vi "Keithley24XX_SR830_Lakeshore336_4Probe_Resistance_Measurement_v2_Controller.vi"() -> ()   [LabVIEW 2018]
uses:
  <instrlib>/Keithley 24XX/Keithley 24XX.lvlib
  <instrlib>/Stanford Research 830/Stanford Research 830.lvlib
  <instrlib>/Lake Shore 336/Lake Shore 336.lvlib
  <instrlib>/Stanford Research 830/Public/Data/Read (All Parameters).vi
  <instrlib>/Keithley 24XX/Public/Data/Read (Single Point).vi
panel:
  in  "Output Level (0)":dbl
  in  "Resistance Manual Range":dbl=1.0
  in  "Current Manual Range":dbl=1.0
  in  "Voltage Manual Range":dbl=1.0
  out "Program Information":string
  out "Front / Rear Terminals":string
  in  "Keithley 24XX Settings":T1(tab)
  out "Enabled Sensing\nFunctions":string
  out "Sensing Current Upper Limit":string
  out "Source Mode:":string
  out "Source Amplitude":dbl
  out "Output Impedence Mode":string
  out "4 Probe Senseing":enum16{"OFF", "ON"}(ring)
  in  "Voltage Auto Range":bool caption="Sync Filter Enabled"
  in  "Current Auto Range":bool caption="Sync Filter Enabled"
  in  "Resistance Auto Range":bool caption="Sync Filter Enabled"
  in  "Update Keithley 24XX GS":bool
  in  "Remote Sensing (4 Wire)":bool
  in  "Displayed Measurement (0: Voltage)":u16(ring)=1 items=["Voltage", "Current", "Resistance"]
  in  "Compliance  Level (0.1)":dbl=0.1
  in  "Source Mode  (0: Voltage)":u16(ring) items=["Voltage", "Current"]
  in  "Output Type  (0: Immediate)":u16(ring) items=["Immediate", "Triggered"]
  out "Output On/Off":bool
  out "Total  Program Iterations":i32
  out "Current Program Iteration":i32
  in  "Program Iterations":i32 min=0 step=1
  out "Channel 1 Display":u16(ring) items=["X", "R", "X Noise", "Aux In 1", "Aux In 2"]
  out "Channel 2 Display":u16(ring) items=["Y", "Theta", "Y Noise", "Aux In 3", "Aux In 4"]
  out "Channel 2\nMeasurement":sgl
  out "Ref\nVoltage (V)":sgl
  out "Channel 1\nMeasurement":sgl
  in  "SR830 Settings":T2(tab)
  out "Channel 1 Display With Ratio":u16(ring) items=["None", "Aux In 1", "Aux In 2"]
  out "Channel 2 Display With Ratio":u16(ring) items=["None", "Aux In 3", "Aux In 4"]
  out "Ref. Amp.":dbl
  out "Ref. Harm.":i32
  out "Ref. Phase":dbl
  out "Trigger Source":u16(ring) items=["Internal", "External"]
  out "Ref. Freq.":dbl
  out "Sensitivity":i16(ring)=-1 items=["Auto Gain"=-1, "2 nV/fA"=0, "5 nV/fA"=1, "10 nV/fA"=2, "20 nV/fA"=3, "50 nV/fA"=4, "100 nV/fA"=5, "200 nV/fA"=6, "500 nV/fA"=7, "1 uV/pA"=8, "2 uV/pA"=9, "5 uV/pA"=10, "10 uV/pA"=11, "20 uV/pA"=12, "50 uV/pA"=13, "100 uV/pA"=14, "200 uV/pA"=15, "500 uV/pA"=16, "1 mV/nA"=17, "2 mV/nA"=18, "5 mV/nA"=19, "10 mV/nA"=20, "20 mV/nA"=21, "50 mV/nA"=22, "100 mV/nA"=23, "200 mV/nA"=24, "500 mV/mA"=25, "1 V/uA"=26]
  out "Time Constant":u16(ring)=8 items=["10 us", "30 us", "100 us", "300 us", "1 ms", "3 ms", "10 ms", "30 ms", "100 ms", "300 ms", "1 s", "3 s", "10 s", "30 s", "100 s", "300 s", "1 ks", "3 ks", "10 ks", "30 ks"]
  out "Low Pass Filter Slope":u16(ring)=1 items=["6 dB/oct", "12 dB/oct", "18 db/oct", "24 dB/oct"]
  out "Input Notch Filter":u16(ring) items=["None", "Line Notch", "2x Line Notch", "Both Notch Filters"]
  out "Dynamic Reserve":i16(ring)=-1 items=["Auto Reserve"=-1, "High Reserve"=0, "Normal"=1, "Low Noise"=2]
  out "Sync Filter Enabled":enum16{"False", "True"}(ring)
  out "Input Shield Grounding":u16(ring) items=["Float", "Ground"]
  out "Input Coupling":u16(ring) items=["AC", "DC"]
  out "Input Connection":u16(ring) items=["Single-Ended Voltage", "Differential Voltage", "1 MOhm Current Gain", "100 MOhm Current Gain"]
  in  "Aquire SR830 GS":bool
  in  "Channel 1 Display With Ratio":u16(ring) items=["None", "Aux In 1", "Aux In 2"]
  in  "Channel 2 Display With Ratio":u16(ring) items=["None", "Aux In 3", "Aux In 4"]
  in  "Channel 1 Display":u16(ring) items=["X", "R", "X Noise", "Aux In 1", "Aux In 2"]
  in  "Channel 2 Display":u16(ring)=1 items=["Y", "Theta", "Y Noise", "Aux In 3", "Aux In 4"]
  in  "Dynamic Reserve":i16(ring)=1 items=["Auto Reserve"=-1, "High Reserve"=0, "Normal"=1, "Low Noise"=2]
  in  "Sensitivity":i16(ring)=17 items=["Auto Gain"=-1, "2 nV/fA"=0, "5 nV/fA"=1, "10 nV/fA"=2, "20 nV/fA"=3, "50 nV/fA"=4, "100 nV/fA"=5, "200 nV/fA"=6, "500 nV/fA"=7, "1 uV/pA"=8, "2 uV/pA"=9, "5 uV/pA"=10, "10 uV/pA"=11, "20 uV/pA"=12, "50 uV/pA"=13, "100 uV/pA"=14, "200 uV/pA"=15, "500 uV/pA"=16, "1 mV/nA"=17, "2 mV/nA"=18, "5 mV/nA"=19, "10 mV/nA"=20, "20 mV/nA"=21, "50 mV/nA"=22, "100 mV/nA"=23, "200 mV/nA"=24, "500 mV/mA"=25, "1 V/uA"=26]
  in  "Sync Filter Enabled":bool
  in  "Low Pass Filter Slope":u16(ring)=1 items=["6 dB/oct", "12 dB/oct", "18 db/oct", "24 dB/oct"]
  in  "Time Constant":u16(ring)=9 items=["10 us", "30 us", "100 us", "300 us", "1 ms", "3 ms", "10 ms", "30 ms", "100 ms", "300 ms", "1 s", "3 s", "10 s", "30 s", "100 s", "300 s", "1 ks", "3 ks", "10 ks", "30 ks"]
  in  "Input Notch Filter (0: None)":u16(ring) items=["None", "Line Notch", "2x Line Notch", "Both Notch Filters"]
  in  "Internal Ref. Freq. (Hz)":dbl=17.0 min=1.0 max=19999.0 step=1.0
  in  "Detection Harmonic Num.":dbl=1.0
  in  "Sine Ref Amplitude (V)":dbl=1.0 min=0.004 max=5.0
  in  "Manual Phase (Degree)":dbl min=-179.99 max=180.0
  in  "Trigger Source":u16(ring) items=["Internal", "External"]
  in  "Input Shield Grounding":u16(ring) items=["Float", "Ground"]
  in  "Input Coupling":u16(ring) items=["AC", "DC"]
  in  "Input Connection":u16(ring)=1 items=["Single-Ended Voltage", "Differential Voltage", "1 MOhm Current Gain", "100 MOhm Current Gain"]
  in  "Update SR830 GS":bool
  in  "Num Steps":i32=1 min=1 step=1
  in  "Total Time (s)":dbl=1.0
  out "Reference Voltage":cluster{u32, dbl}[](graph)
  out "Step Size (V)":dbl=1.0 min=0.004 max=5.0
  in  "Start Output Amplitude (V)":dbl=1.0 min=0.004 max=5.0
  in  "Final Output Amplitude (V)":dbl=1.0 min=0.004 max=5.0
  out "Step Time (ms)":dbl=50.0
  in  "Idle Measuring Time (ms)":i32=500
  out "VI State":T3(ring)
  in  "Idle Measure\nLakeShore 336 \nStatus":bool=TRUE
  in  "Idle Measure \nKeithley 24XX\nStatus":bool=TRUE
  in  "Idle Measure\nSR830 Status":bool=TRUE
  in  "Lakeshore 366\nVISA resource name":refnum<visa-resource-name>="GPIB0::12::INSTR"
  in  "Lakeshore Initialized / Off":bool
  in  "Reset LakeShore\non Initialize":bool
  in  "Keithley24XX Gate\nVISA resource name":refnum<visa-resource-name>="GPIB0::23::INSTR" caption="Keithley 24XX Gate\nVISA resource name"
  in  "Keithley 24XX Initialized / Off":bool
  in  "Reset Keithley\non Initialize":bool
  in  "SR830 Initialized / Off":bool
  in  "Reset SR830\non Initialize":bool
  in  "SR830\nVISA resource name":refnum<visa-resource-name>="GPIB0::8::INSTR" caption="SR830 VISA \nresource name"
  out "Theta : XYGraph":cluster{"Y":dbl[], "Y":dbl[]}[](graph)
  out "Temp : XYGraph":cluster{"Y":dbl[], "Y":dbl[]}[](graph)
  out "Resistance : XYGraph":cluster{"Y":dbl[], "Y":dbl[]}[](graph)
  out "I_leak : XYGraph":cluster{"Y":dbl[], "Y":dbl[]}[](graph)
  out "Resistance / Differential":bool
  out "Gate Voltage":bool
  in  "Temperature":bool
  in  "Phase":bool
  in  "Gate Leakage Current":bool
  out "Dup path":path
  in  "<File Name>.txt (Don't add extension)":string
  in  "Data Save Path:":path=path "C:/Users/labpc/Documents/ProbeStation Users Data"
  in  "Measurement Output":T4(radio)
  in  "Series Resistance (Ohms)\n[Apparatus Constant]":dbl=10000000.0 format="%_6e"
  in  "Measurement \nDelay Time (s)":dbl=30.0
  in  "Source Voltage\nStep Time (ms)\n 4Probe":dbl=20.0
  in  "Source Voltage\nStep Size (V) \n4Probe":dbl=0.01
  in  "Source Measurement Voltage (V)":dbl=1.0
  in  "Source Voltage \nWarmup Delay \n(Before Gating)":bool
  in  "Source Voltage\nRamp On/Off":bool
  in  "Source Voltage\nStep Time (ms)":dbl=200.0
  in  "Source Voltage\nStep Size (V)":dbl=0.05
  in  "Source Voltage\nFinal (V)":dbl
  in  "Source Voltage\nInitial (V)":dbl
  out "Measured Gate\nVoltage (V)":sgl
  out "Gate leakage \ncurrent (A)":sgl
  in  "Gate\nMeasure":bool
  in  "Gate \nStep Time (ms)":dbl=200.0
  in  "Gate\nStep Time (ms)":dbl=200.0
  in  "Gate Voltage\nStep Size (V)":dbl=0.05
  in  "Gate \nVoltage Final (V)":dbl
  in  "Low Gate \nVoltage (V)":dbl=-80.0
  in  "Gate Voltage\nInitial Traversal Direction":enum16{"Upward", "Downward"}(ring)
  in  "Gate Voltage \nStep Size (V)":dbl=0.1
  in  "High Gate \nVoltage (V)":dbl=80.0
  in  "Gate Voltage\nInitial (V)":dbl
  in  "Gate\nReset":bool
  in  "Gate Current\nCompliance Level (A)":dbl=1.0000000005838672e-07
  in  "Run Program":bool
  in  "Stop VI":bool
  in  "Program Selection":T5(radio)
  # "Welcome to Matt Gebert's Keithley / SR830 / Lakeshore 4 Probe Measurement Controller. This Labview program controls the configuration and measurements of one Keithelys 24XX, one SR830 and one LakeShore Controller, through a state machine architecture.\nIf using sensitive samples, be careful of \"rsetting\" equipment, due to fluctuations of output signals. \"General settings\" tabs will be applied at the start of a measurement program, or by being manually applied (button on page).\nPrograms written allow:\n   1) Ramp voltages to initial points for measurements.     2) Perform a 4 Probe DC Gate measurement using the Keithley & SR830."
  # "Sensing Configuration"
  # "Program: Ramp Gate Voltage Configuration"
  # "Program Control"
  # "Program: 4 Probe Measurement Configuration"
  # "Input Configuration"
  # "Measurement Configuration"
  # "Reference Configuration"
  # "Channel Displays"
  # "Channel Displays"
  # "Reference Configuration"
  # "Input Configuration"
  # "Measurement Configuration"
  # "Ramps source voltage to avoid damaging samples.\nNote the current Ref Voltage above if you are in the \"Idle\" state."
  # "4 Probe Output Configuration"
  # "Recorded Params"
  # "Output Data"
  # "Program: 4 Probe Measurement Configuration"
  # "Program: Ramp Source Voltage Configuration"
  # "SR830 Source\n& Meas. Control"
  # "Keithley Gate\nVoltage Control"
  # "LakeShore 336 \nTemperature \nController"
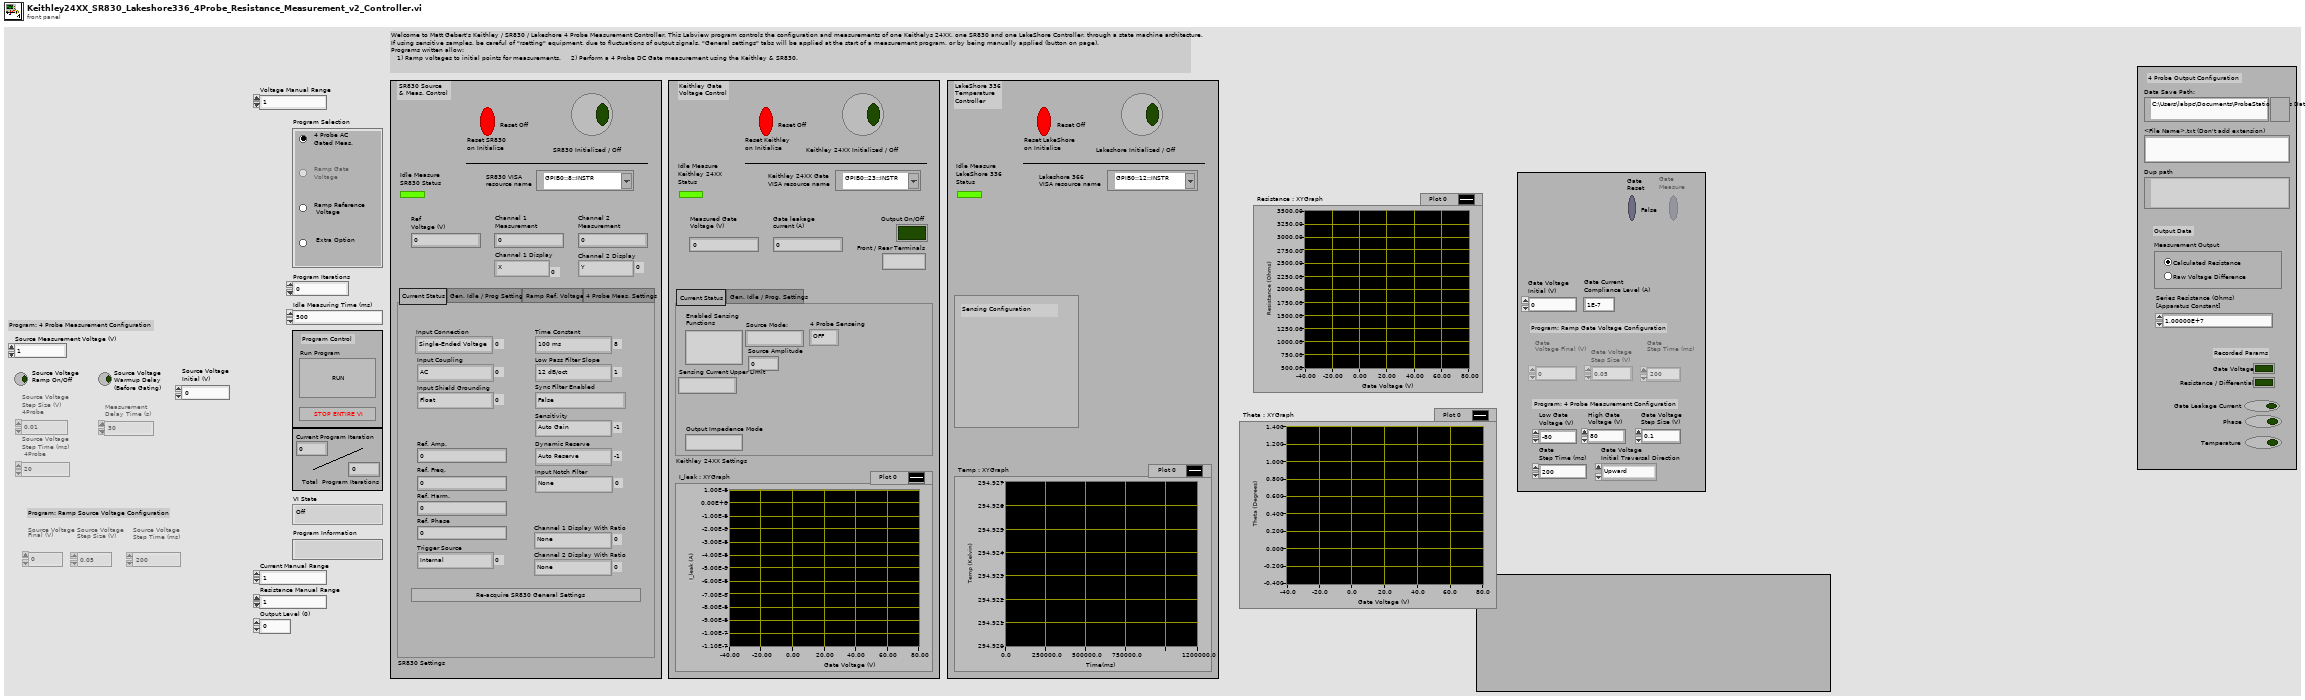
[diagram p1: front panel]
types:
  T1 = enum32{"Current Status", "Gen. Idle / Prog. Settings"}
  T2 = enum32{"Current Status", "Gen. Idle / Prog Settings", "Ramp Ref. Voltage", "4 Probe Meas. Settings"}
  T3 = enum16{"Off", "Idle | Waiting for event", "Running single meas.", "Running multi meas.", "Running continuous meas."}
  T4 = enum32{"Calculated Resistance", "Raw Voltage Difference"}
  T5 = enum32{"4 Probe Gated Measurement", "Ramp Gate Voltage", "Ramp Ref Voltage", "Extra Option"}
  T6 = enum32{"Current Status", "Gen. Idle / Prog. Settings", "Ramp Ref. Voltage", "4 Probe Meas. Settings"}
  T7 = cluster{"Lakeshore 366 VISA Name":refnum<visa-resource-name>, "Lakeshore Error":errorcluster, "Keithley 24XX VISA Name":refnum<visa-resource-name>, "Keithley 24XX Error":errorcluster, "SR830 VISA Name":refnum<visa-resource-name>, "SR830 Error":errorcluster, "MeasurementsRemaining":i32, "TotalMeasurements":i32}
  T8 = cluster{"Baud Rate":u32, "Parity":u16, "Data Bits":u16, "Stop Bits":u16, "Flow Control":u16}
  T9 = cluster{"X-Value":dbl, "Y-Value":dbl, "R-Value":dbl, "Theta-Value":dbl, "Aux In 1 Value":dbl, "Aux In 2 Value":dbl, "Aux In 3 Value":dbl, "Aux In 4 Value":dbl, "Reference Frequency":dbl, "Channel 1 Display":dbl, "Channel 2 Display":dbl}
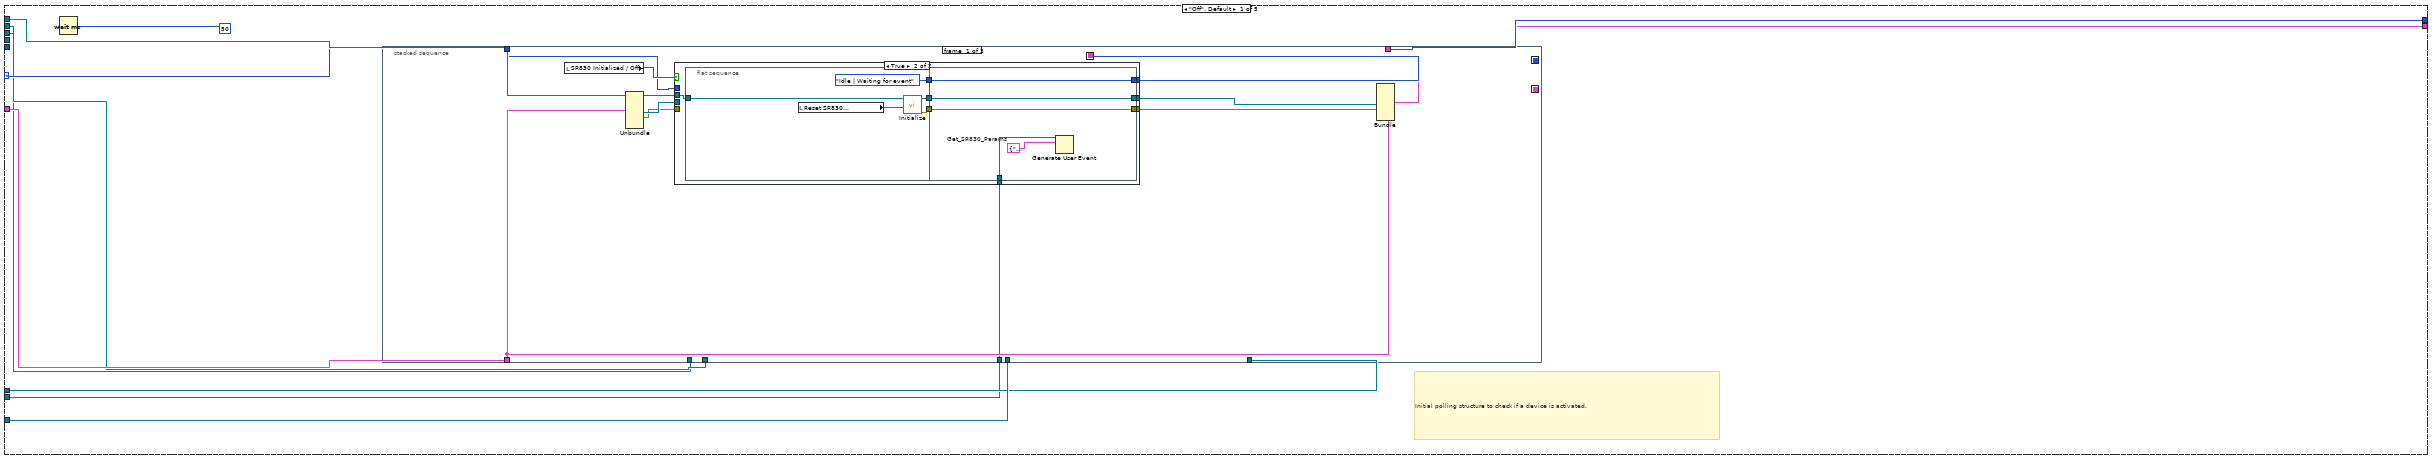
[diagram p7: hidden frame]
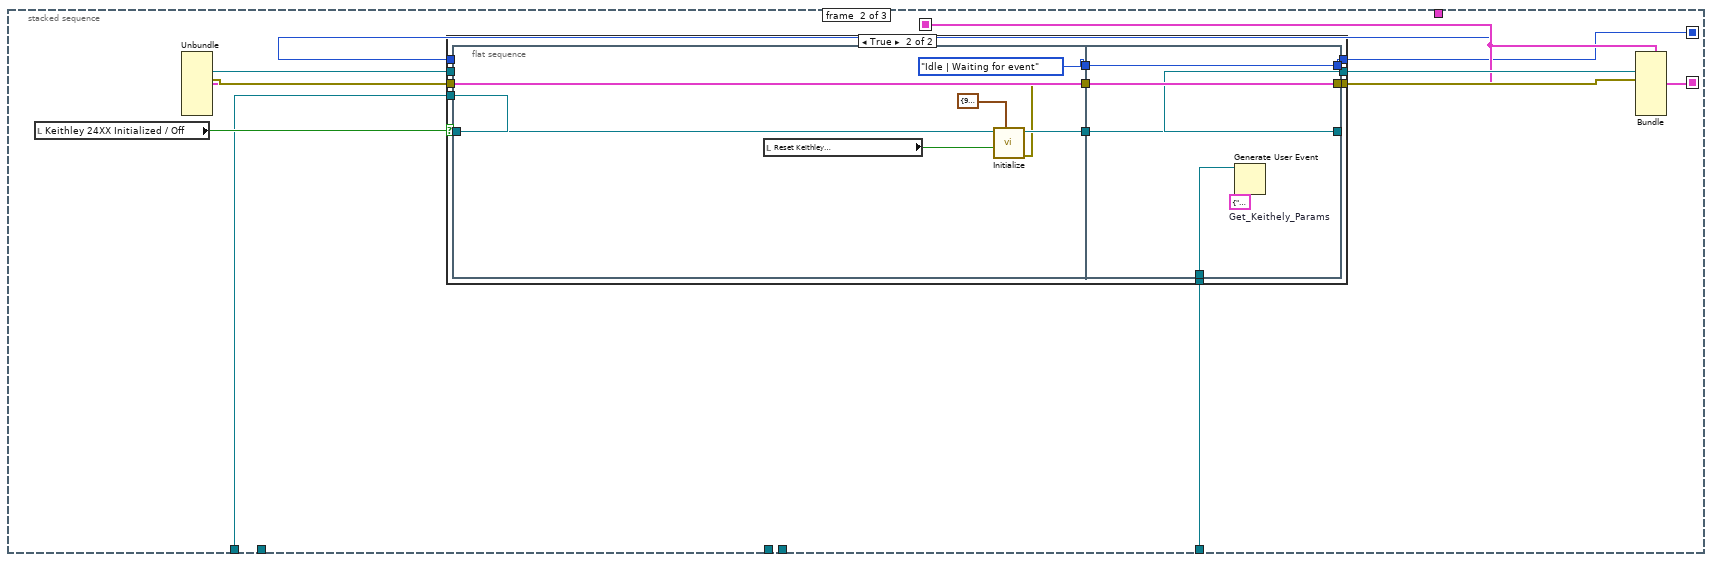
[diagram p9: hidden frame]
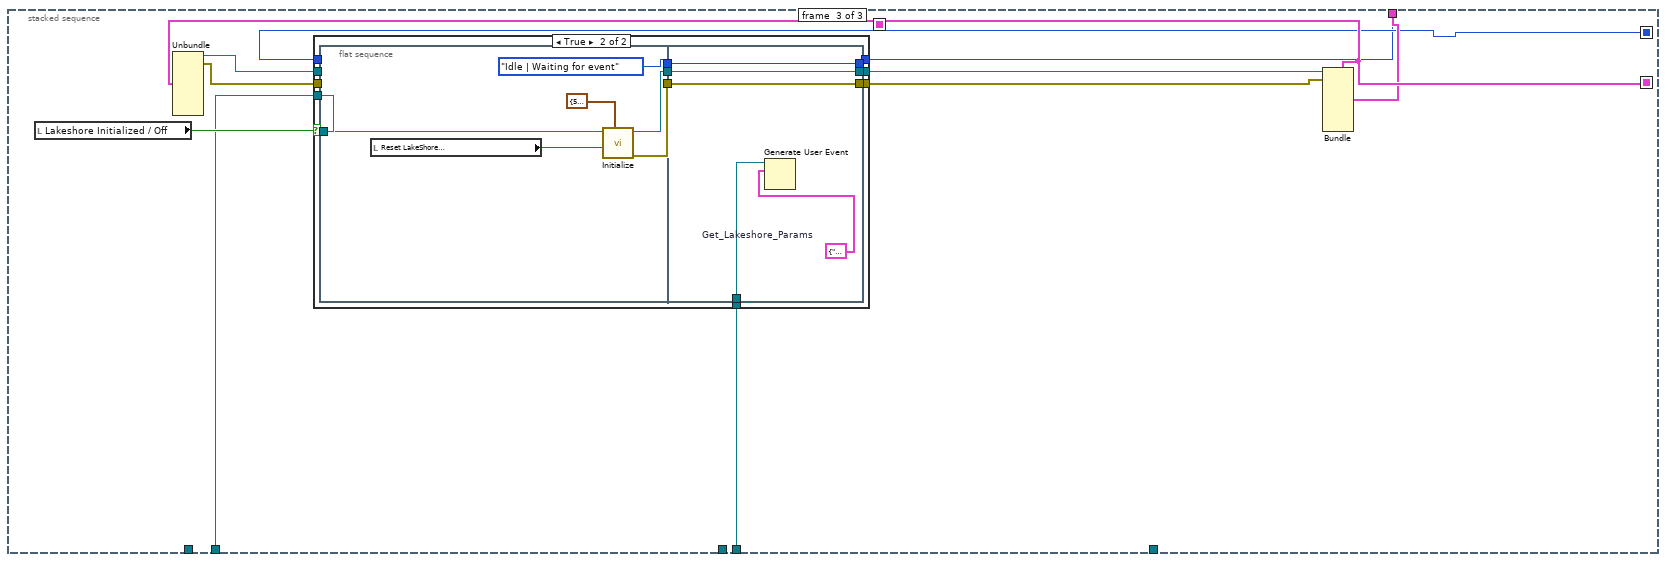
[diagram p11: hidden frame]
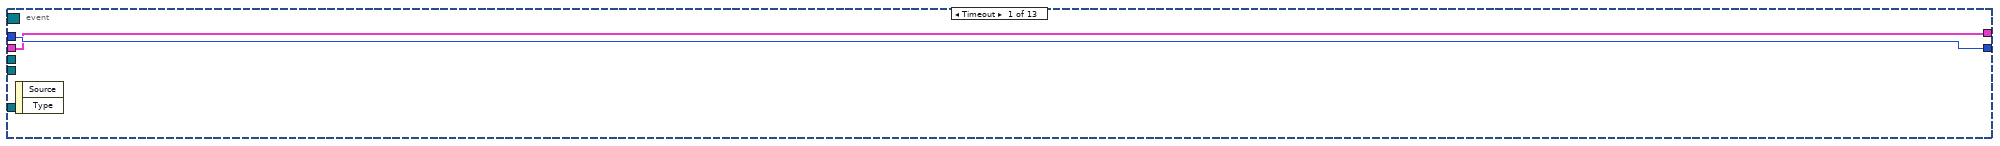
[diagram p13: hidden frame]
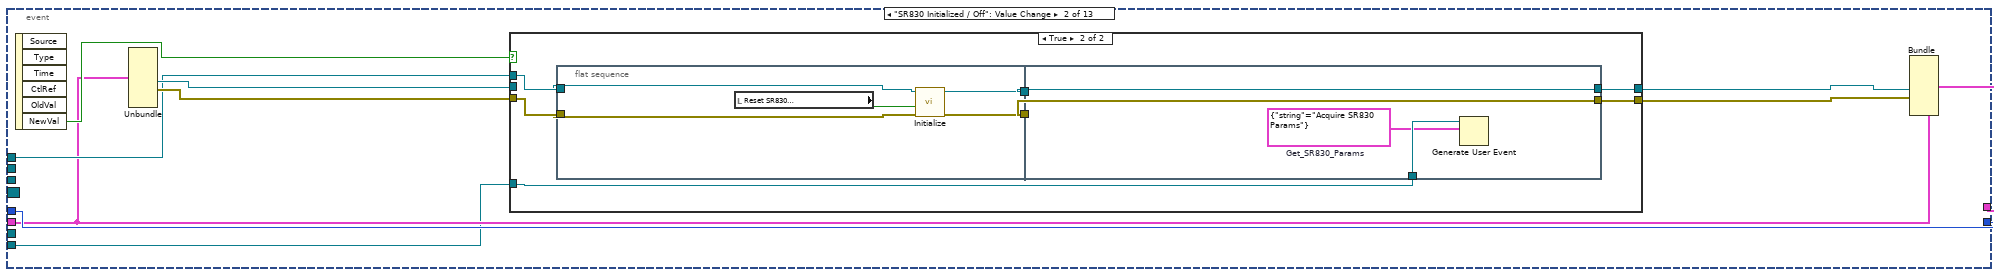
[diagram p14: hidden frame]
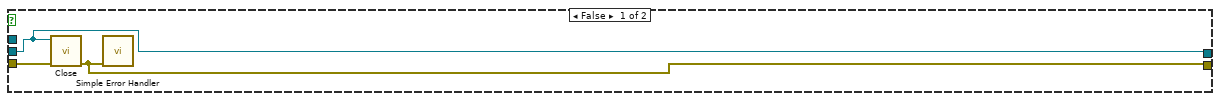
[diagram p15: hidden frame]
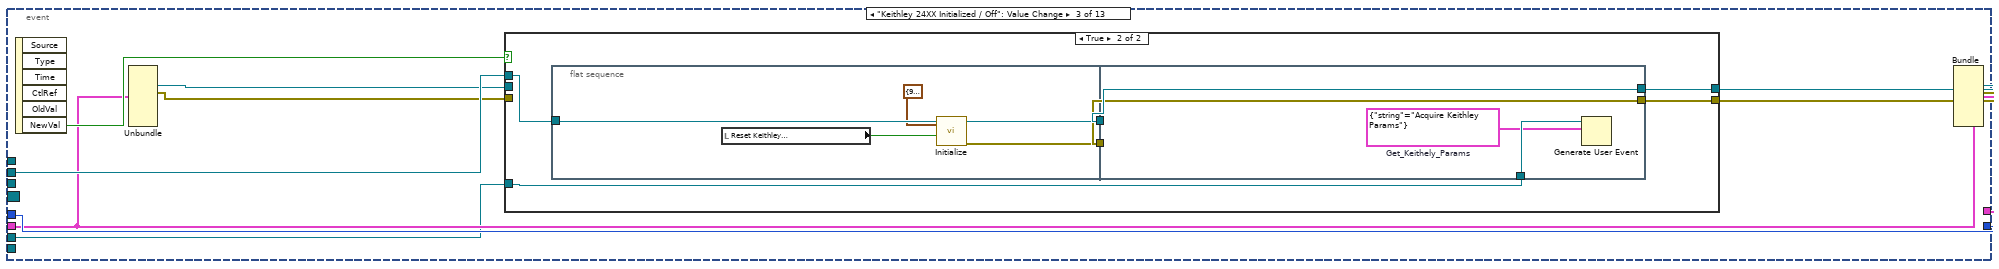
[diagram p16: hidden frame]
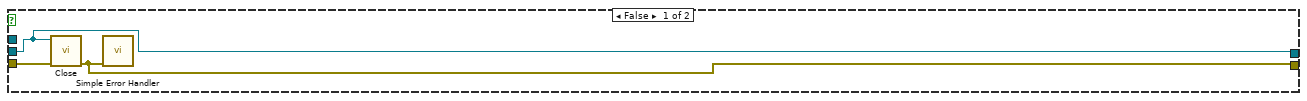
[diagram p17: hidden frame]
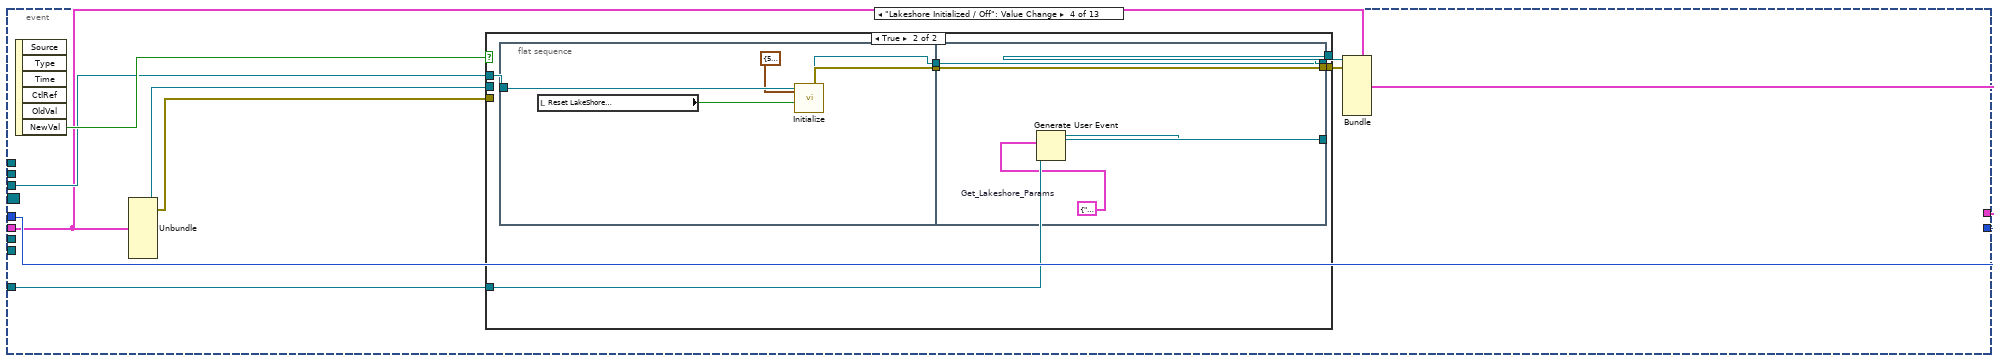
[diagram p18: hidden frame]
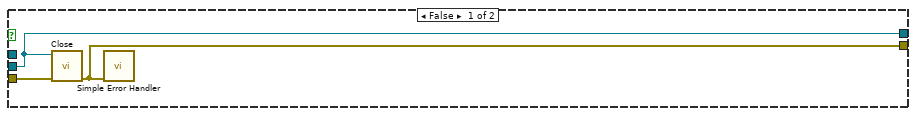
[diagram p19: hidden frame]
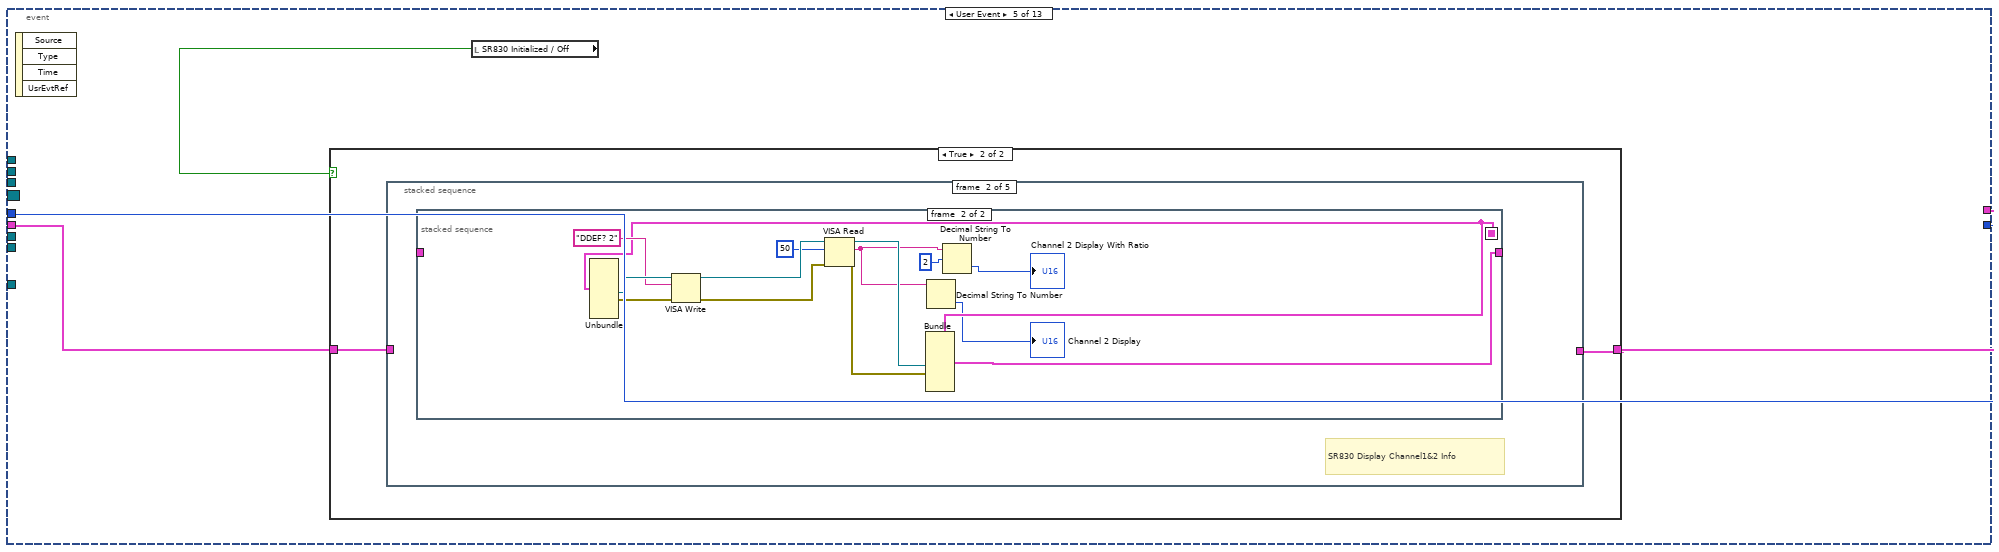
[diagram p20: hidden frame]
diagram:
  w7 = cluster{"string":string} {"string"="Acquire Lakeshore Params"}  # Get_Lakeshore_Params
  w4 = cluster{"string":string} {"string"="Acquire SR830 Params"}  # Get_SR830_Params
  w8 = cluster{"string":string} {"string"="Acquire Keithley Params"}  # Get_Keithely_Params
  w9 = cluster{"string":string} {"string"="UI Update"}  # UI Update
  (unwired) T6."Current Status" ("SR830 Settings")
  w12 = FALSE ("Lakeshore Initialized / Off")
  w19 = TRUE ("Gate Voltage")
  # "TODO: \n1. Make resource error checking mechanism for programs and Idle loop.\n2. Figure out why exiting loop doesn't display generated errors...\n4. Add radio buttons for a) continuous, b) multiple, c) single measurements\n3. UI updates for changing \"Program Selection\" value. Ie, which measurement types are allowed.\n4. UI Updates for enabling / disabling resources\n5. Program event data changes for ramping"
  # "Ensure devices are disconnected on program exit, if \"stopped\"."
  n1 = local read "SR830 Settings"() -> ()  [unwired: 1 in]
  n2 = Create User Event(user event datatype=w9) -> (user event=w5:refnum<user-event>)  [unwired: 1 in, 1 out]
  n3 = Create User Event(user event datatype=w7) -> (user event=w1:refnum<user-event>)  [unwired: 1 in, 1 out]
  n4 = Create User Event(user event datatype=w8) -> (user event=w2:refnum<user-event>)  [unwired: 1 in, 1 out]
  n5 = Create User Event(user event datatype=w4) -> (user event=w3:refnum<user-event>)  [unwired: 1 in, 1 out]
  n6 = register-events(w5, w2, w3, w1) -> (reference out=w6:refnum<event-registration>)  [unwired: 2 in, 1 out]
  n7 = local write "SR830 Initialized / Off"(w12) -> ()
  n8 = local write "Keithley 24XX Initialized / Off"(w12) -> ()
  n9 = local write "Lakeshore Initialized / Off"(w12) -> ()
  n10 = while {
    shift-right: [w29] -> w15
    shift-left: T3."Off" -> [w32]
    shift-right: [w25] -> w13
    shift-left: T7 {"Lakeshore 366 VISA Name"="", "Lakeshore Error"={"status"=FALSE, "code"=0, "source"=""}, "Keithley 24XX VISA Name"="", "Keithley 24XX Error"={"status"=FALSE, "code"=0, "source"=""}, "SR830 VISA Name"="", "SR830 Error"={"status"=FALSE, "code"=0, "source"=""}, "MeasurementsRemaining"=0, "TotalMeasurements"=0} -> [w26]
    tunnel: "Program Selection" -> [w24]
    tunnel: w6 -> [w23]
    tunnel: w3 -> [w22]
    tunnel: w2 -> [w21]
    tunnel: w1 -> [w20]
    stop <- "Stop VI" stop-if-true
    # "State Machine"
    n11 = local read "Keithley24XX Gate\nVISA resource name"() -> (w31:refnum<visa-resource-name>)
    n12 = local read "Lakeshore 366\nVISA resource name"() -> (w30:refnum<visa-resource-name>)
    n13 = local read "SR830\nVISA resource name"() -> (w27:refnum<visa-resource-name>)
    n14 = case shown="\"Idle | Waiting for event\"" w32 {
      selector: w32 -> [w42 w158 _ w908 w918]
      tunnel: w31 -> [w37 w153 _ _ _]
      tunnel: w30 -> [w38 w155 _ _ _]
      tunnel: [w41 w157 T3."Idle | Waiting for event" w907 w918] -> w29
      tunnel: w27 -> [w43 w154 _ _ _]
      tunnel: w26 -> [w40 w152 w878 w910 w917]
      tunnel: [w39 w147 w879 w904 w917] -> w25
      tunnel: w24 -> [_ _ w880 _ _]
      tunnel: w23 -> [_ w145 _ _ _]
      tunnel: w22 -> [w33 w144 _ _ _]
      tunnel: w21 -> [w34 w143 _ _ _]
      tunnel: w20 -> [w35 w142 _ _ _]
      frame "Off", Default {
        # "Initial polling structure to check if a device is activated."
        n15 = Wait (ms)(milliseconds to wait=u32 50) -> ()  [unwired: 1 out]
        n16 = stacked-sequence {
          seq-local: [w47 _ _] -> [_ w81 _]
          seq-local: [w45 _ _] -> [_ w82 _]
          seq-local: [_ w80 _] -> [_ _ w111]
          seq-local: [_ w78 _] -> [_ _ w114]
          tunnel: w43 -> [w49 _ _]
          tunnel: w42 -> [w48 _ _]
          tunnel: w40 -> [w46 _ _]
          tunnel: w37 -> [_ w77 _]
          tunnel: [_ _ w110] -> w41
          tunnel: [_ _ w113] -> w39
          tunnel: w38 -> [_ _ w112]
          tunnel: w35 -> [_ _ w109]
          tunnel: w34 -> [_ w76 _]
          tunnel: w33 -> [w44 _ _]
          frame #0 {
            n17 = local read "SR830 Initialized / Off"() -> (w54:bool)
            n18 = Unbundle(w46) -> ("SR830 VISA Name"=w51:refnum<visa-resource-name>, "SR830 Error"=w50:errorcluster)  [unwired: 6 out]
            n19 = case shown="True" w54 {
              tunnel: w49 -> [_ w65]
              tunnel: [w57 w64] -> w53
              tunnel: [w55 w63] -> w52
              tunnel: w51 -> [w57 _]
              tunnel: w50 -> [w55 _]
              tunnel: w48 -> [w56 _]
              tunnel: [w56 w62] -> w47
              tunnel: w44 -> [_ w58]
              frame False {
              }
              frame True {
                n20 = flat-sequence {
                  tunnel: w65 -> [w70]
                  tunnel: [w69] -> w61
                  tunnel: [w68] -> w60
                  tunnel: [T3."Idle | Waiting for event"] -> w59
                  tunnel: [w73] -> w62
                  tunnel: [w74] -> w63
                  tunnel: [w75] -> w64
                  tunnel: w61 -> [w75]
                  tunnel: w60 -> [w74]
                  tunnel: w59 -> [w73]
                  tunnel: w58 -> [w71]
                  frame #0 {
                    n21 = local read "Reset SR830\non Initialize"() -> (w67:bool)
                    n22 = call <instrlib>:"Initialize.vi"("Reset (True)"=w67, "VISA resource name"=w70) -> ("error out"=w68:errorcluster, "VISA resource name out"=w69:refnum<visa-resource-name>)  [unwired: 8 in]
                  }
                  frame #1 {
                    w72 = cluster{"string":string} {"string"="Acquire SR830 Params"}  # Get_SR830_Params
                    n23 = Generate User Event(user event=w71, event data cluster=w72) -> ()  [unwired: 2 in, 2 out]
                  }
                }
              }
            }
            n24 = Bundle(cluster=w46, "SR830 VISA Name"=w53, "SR830 Error"=w52) -> (w45:T7)  [unwired: 6 in]
          }
          frame #1 {
            n25 = local read "Keithley 24XX Initialized / Off"() -> (w79:bool)
            n26 = Unbundle(w82) -> ("Keithley 24XX VISA Name"=w83:refnum<visa-resource-name>, "Keithley 24XX Error"=w84:errorcluster)  [unwired: 6 out]
            n27 = case shown="True" w79 {
              tunnel: [w87 w96] -> w86
              tunnel: [w89 w97] -> w85
              tunnel: w83 -> [w89 _]
              tunnel: w84 -> [w87 _]
              tunnel: [w88 w95] -> w80
              tunnel: w81 -> [w88 _]
              tunnel: w77 -> [_ w94]
              tunnel: w76 -> [_ w90]
              frame False {
              }
              frame True {
                n28 = flat-sequence {
                  tunnel: w94 -> [w98]
                  tunnel: [w103] -> w93
                  tunnel: [w102] -> w92
                  tunnel: [T3."Idle | Waiting for event"] -> w91
                  tunnel: [w106] -> w95
                  tunnel: [w107] -> w96
                  tunnel: [w108] -> w97
                  tunnel: w93 -> [w108]
                  tunnel: w92 -> [w107]
                  tunnel: w91 -> [w106]
                  tunnel: w90 -> [w104]
                  frame #0 {
                    n29 = local read "Reset Keithley\non Initialize"() -> (w100:bool)
                    n30 = call <instrlib>:"Initialize.vi"("Serial Configuration"=T8 {"Baud Rate"=9600, "Parity"=0, "Data Bits"=8, "Stop Bits"=10, "Flow Control"=0}, "Reset (True)"=w100, "VISA resource name"=w98) -> ("error out"=w102:errorcluster, "VISA resource name out"=w103:refnum<visa-resource-name>)  [unwired: 7 in]
                  }
                  frame #1 {
                    w105 = cluster{"string":string} {"string"="Acquire Keithley Params"}  # Get_Keithely_Params
                    n31 = Generate User Event(user event=w104, event data cluster=w105) -> ()  [unwired: 2 in, 2 out]
                  }
                }
              }
            }
            n32 = Bundle(cluster=w82, "Keithley 24XX VISA Name"=w85, "Keithley 24XX Error"=w86) -> (w78:T7)  [unwired: 6 in]
          }
          frame #2 {
            n33 = local read "Lakeshore Initialized / Off"() -> (w115:bool)
            n34 = Unbundle(w114) -> ("Lakeshore 366 VISA Name"=w116:refnum<visa-resource-name>, "Lakeshore Error"=w117:errorcluster)  [unwired: 6 out]
            n35 = case shown="True" w115 {
              tunnel: [w121 w130] -> w119
              tunnel: [w122 w129] -> w118
              tunnel: w116 -> [w122 _]
              tunnel: w117 -> [w121 _]
              tunnel: [w120 w128] -> w110
              tunnel: w112 -> [_ w127]
              tunnel: w111 -> [w120 _]
              tunnel: w109 -> [_ w123]
              frame False {
              }
              frame True {
                n36 = flat-sequence {
                  tunnel: w127 -> [w131]
                  tunnel: [w135] -> w126
                  tunnel: [w134] -> w125
                  tunnel: [T3."Idle | Waiting for event"] -> w124
                  tunnel: [w139] -> w128
                  tunnel: [w140] -> w129
                  tunnel: [w141] -> w130
                  tunnel: w126 -> [w141]
                  tunnel: w125 -> [w140]
                  tunnel: w124 -> [w139]
                  tunnel: w123 -> [w137]
                  frame #0 {
                    n37 = local read "Reset LakeShore\non Initialize"() -> (w133:bool)
                    n38 = call <instrlib>:"Initialize.vi"("Serial Configuration"=T8 {"Baud Rate"=57600, "Parity"=1, "Data Bits"=7, "Stop Bits"=10, "Flow Control"=0}, "Reset (True)"=w133, "VISA resource name"=w131) -> ("error out"=w135:errorcluster, "VISA resource name out"=w134:refnum<visa-resource-name>)  [unwired: 7 in]
                  }
                  frame #1 {
                    w138 = cluster{"string":string} {"string"="Acquire Lakeshore Params"}  # Get_Lakeshore_Params
                    n39 = Generate User Event(user event=w137, event data cluster=w138) -> ()  [unwired: 2 in, 2 out]
                  }
                }
              }
            }
            n40 = Bundle(cluster=w114, "Lakeshore 366 VISA Name"=w118, "Lakeshore Error"=w119) -> (w113:T7)  [unwired: 6 in]
          }
        }
      }
      frame "Idle | Waiting for event" {
        n41 = flat-sequence {
          tunnel: w158 -> [w170]
          tunnel: [w169] -> w156
          tunnel: w155 -> [w168]
          tunnel: w154 -> [w167]
          tunnel: w153 -> [w166]
          tunnel: w152 -> [w165]
          tunnel: [w164] -> w148
          tunnel: w145 -> [w162]
          tunnel: w144 -> [w161]
          tunnel: w143 -> [w160]
          tunnel: w142 -> [w159]
          tunnel: w156 -> [w804]
          tunnel: [w805] -> w151
          tunnel: [w803] -> w150
          tunnel: [w802] -> w149
          tunnel: [w801] -> w146
          tunnel: [w815] -> w157
          tunnel: w151 -> [w815]
          tunnel: w150 -> [w811]
          tunnel: w149 -> [w810]
          tunnel: w148 -> [w814]
          tunnel: [w813] -> w147
          tunnel: w146 -> [w812]
          frame #0 {
            n42 = event shown="[11] \"Update Keithley 24XX GS\": Mouse Up" {
              selector: w162 -> [_ _ _ _ _ _ _ _ _ _ _ _ _]
              dyn-events: _ -> [_ _ _ _ _ _ _ _ _ _ _ _ _]
              timeout: "Idle Measuring Time (ms)" -> [_ _ _ _ _ _ _ _ _ _ _ _ _]
              tunnel: w170 -> [w172 w176 w205 w238 w258 w481 w584 w586 w588 _ w612 w715 w793]
              tunnel: [w172 w176 w205 w238 w258 w481 w584 w586 w588 w591 w612 w715 w793] -> w169
              tunnel: w168 -> [_ _ _ w237 _ _ _ _ _ _ _ _ _]
              tunnel: w167 -> [_ w177 _ _ _ _ _ _ _ _ _ _ _]
              tunnel: w166 -> [_ _ w210 _ _ _ _ _ _ _ _ _ _]
              tunnel: w165 -> [w171 w175 w204 w232 w261 w483 w585 w587 w589 w595 w615 w714 w792]
              tunnel: [w171 w174 w203 w231 w259 w482 w585 w587 w589 w594 w616 w713 w792] -> w164
              tunnel: w161 -> [_ w173 _ _ _ _ _ _ _ _ _ _ _]
              tunnel: w160 -> [_ _ w202 _ _ _ _ _ _ _ _ _ _]
              tunnel: w159 -> [_ _ _ w230 _ _ _ _ _ _ _ _ _]
              event Timeout {
                n43 = event-data() -> ()  [unwired: 1 in, 2 out]
              }
              event "SR830 Initialized / Off": Value Change {
                n44 = event-data() -> ("NewVal"=w182:bool)  [unwired: 1 in, 5 out]
                n45 = Unbundle(w175) -> ("SR830 VISA Name"=w181:refnum<visa-resource-name>, "SR830 Error"=w180:errorcluster)  [unwired: 6 out]
                n46 = case shown="True" w182 {
                  tunnel: w181 -> [w183 _]
                  tunnel: w180 -> [w185 w191]
                  tunnel: [w184 w190] -> w179
                  tunnel: [w183 w189] -> w178
                  tunnel: w177 -> [_ w192]
                  tunnel: w173 -> [_ w186]
                  frame False {
                    n47 = call <instrlib>:"Close.vi"("error in (no error)"=w185, "VISA resource name"=w183) -> ("error out"=w184:errorcluster)  [unwired: 9 in]
                    n48 = call <vilib>:"Simple Error Handler.vi"("error in (no error)"=w184) -> ()  [unwired: 4 in, 5 out]
                  }
                  frame True {
                    n49 = flat-sequence {
                      tunnel: w192 -> [w197]
                      tunnel: w191 -> [w196]
                      tunnel: [w195] -> w188
                      tunnel: [w194] -> w187
                      tunnel: [w200] -> w189
                      tunnel: [w201] -> w190
                      tunnel: w188 -> [w201]
                      tunnel: w187 -> [w200]
                      tunnel: w186 -> [w199]
                      frame #0 {
                        n50 = local read "Reset SR830\non Initialize"() -> (w193:bool)
                        n51 = call <instrlib>:"Initialize.vi"("error in (no error)"=w196, "Reset (True)"=w193, "VISA resource name"=w197) -> ("error out"=w195:errorcluster, "VISA resource name out"=w194:refnum<visa-resource-name>)  [unwired: 7 in]
                      }
                      frame #1 {
                        w198 = cluster{"string":string} {"string"="Acquire SR830 Params"}  # Get_SR830_Params
                        n52 = Generate User Event(user event=w199, event data cluster=w198) -> ()  [unwired: 2 in, 2 out]
                      }
                    }
                  }
                }
                n53 = Bundle(cluster=w175, "SR830 VISA Name"=w178, "SR830 Error"=w179) -> (w174:T7)  [unwired: 6 in]
              }
              event "Keithley 24XX Initialized / Off": Value Change {
                n54 = event-data() -> ("NewVal"=w211:bool)  [unwired: 1 in, 5 out]
                n55 = Unbundle(w204) -> ("Keithley 24XX VISA Name"=w207:refnum<visa-resource-name>, "Keithley 24XX Error"=w206:errorcluster)  [unwired: 6 out]
                n56 = case shown="True" w211 {
                  tunnel: w210 -> [_ w220]
                  tunnel: [w213 w219] -> w209
                  tunnel: [w212 w218] -> w208
                  tunnel: w207 -> [w213 _]
                  tunnel: w206 -> [w214 _]
                  tunnel: w202 -> [_ w215]
                  frame False {
                    n57 = call <instrlib>:"Close.vi"("error in (no error)"=w214, "VISA resource name"=w213) -> ("error out"=w212:errorcluster)  [unwired: 9 in]
                    n58 = call <vilib>:"Simple Error Handler.vi"("error in (no error)"=w212) -> ()  [unwired: 4 in, 5 out]
                  }
                  frame True {
                    n59 = flat-sequence {
                      tunnel: w220 -> [w225]
                      tunnel: [w224] -> w217
                      tunnel: [w223] -> w216
                      tunnel: [w228] -> w218
                      tunnel: [w229] -> w219
                      tunnel: w217 -> [w229]
                      tunnel: w216 -> [w228]
                      tunnel: w215 -> [w227]
                      frame #0 {
                        n60 = local read "Reset Keithley\non Initialize"() -> (w222:bool)
                        n61 = call <instrlib>:"Initialize.vi"("Serial Configuration"=T8 {"Baud Rate"=9600, "Parity"=0, "Data Bits"=8, "Stop Bits"=10, "Flow Control"=0}, "Reset (True)"=w222, "VISA resource name"=w225) -> ("error out"=w223:errorcluster, "VISA resource name out"=w224:refnum<visa-resource-name>)  [unwired: 7 in]
                      }
                      frame #1 {
                        w226 = cluster{"string":string} {"string"="Acquire Keithley Params"}  # Get_Keithely_Params
                        n62 = Generate User Event(user event=w227, event data cluster=w226) -> ()  [unwired: 2 in, 2 out]
                      }
                    }
                  }
                }
                n63 = Bundle(cluster=w204, "Keithley 24XX VISA Name"=w209, "Keithley 24XX Error"=w208) -> (w203:T7)  [unwired: 6 in]
              }
              event "Lakeshore Initialized / Off": Value Change {
                n64 = event-data() -> ("NewVal"=w239:bool)  [unwired: 1 in, 5 out]
                n65 = Unbundle(w232) -> ("Lakeshore 366 VISA Name"=w236:refnum<visa-resource-name>, "Lakeshore Error"=w235:errorcluster)  [unwired: 6 out]
                n66 = case shown="True" w239 {
                  tunnel: w237 -> [_ w248]
                  tunnel: w236 -> [w241 _]
                  tunnel: w235 -> [w242 _]
                  tunnel: [w241 w246] -> w234
                  tunnel: [w240 w247] -> w233
                  tunnel: w230 -> [_ w243]
                  frame False {
                    n67 = call <instrlib>:"Close.vi"("error in (no error)"=w242, "VISA resource name"=w241) -> ("error out"=w240:errorcluster)  [unwired: 9 in]
                    n68 = call <vilib>:"Simple Error Handler.vi"("error in (no error)"=w240) -> ()  [unwired: 4 in, 5 out]
                  }
                  frame True {
                    n69 = flat-sequence {
                      tunnel: w248 -> [w253]
                      tunnel: [w252] -> w245
                      tunnel: [w251] -> w244
                      tunnel: [w256] -> w246
                      tunnel: [w257] -> w247
                      tunnel: w245 -> [w257]
                      tunnel: w244 -> [w256]
                      tunnel: w243 -> [w254]
                      frame #0 {
                        n70 = local read "Reset LakeShore\non Initialize"() -> (w250:bool)
                        n71 = call <instrlib>:"Initialize.vi"("Serial Configuration"=T8 {"Baud Rate"=57600, "Parity"=1, "Data Bits"=7, "Stop Bits"=10, "Flow Control"=0}, "Reset (True)"=w250, "VISA resource name"=w253) -> ("error out"=w252:errorcluster, "VISA resource name out"=w251:refnum<visa-resource-name>)  [unwired: 7 in]
                      }
                      frame #1 {
                        w255 = cluster{"string":string} {"string"="Acquire Lakeshore Params"}  # Get_Lakeshore_Params
                        n72 = Generate User Event(user event=w254, event data cluster=w255) -> ()  [unwired: 2 in, 2 out]
                      }
                    }
                  }
                }
                n73 = Bundle(cluster=w232, "Lakeshore 366 VISA Name"=w234, "Lakeshore Error"=w233) -> (w231:T7)  [unwired: 6 in]
              }
              event User Event {
                n74 = event-data() -> ()  [unwired: 1 in, 4 out]
                n75 = local read "SR830 Initialized / Off"() -> (w260:bool)
                n76 = case shown="True" w260 {
                  tunnel: [w262 w263] -> w259
                  tunnel: w261 -> [w262 w264]
                  frame False {
                  }
                  frame True {
                    n77 = stacked-sequence {
                      seq-local: [w265 _ _ _ _] -> [_ w331 _ _ _]
                      seq-local: [_ w330 _ _ _] -> [_ _ w361 _ _]
                      seq-local: [_ _ w360 _ _] -> [_ _ _ w411 _]
                      seq-local: [_ _ _ w410 _] -> [_ _ _ _ w475]
                      tunnel: w264 -> [w266 _ _ _ _]
                      tunnel: [_ _ _ _ w474] -> w263
                      frame #0 {
                        # "SR830 Reference Information"
                        n78 = stacked-sequence {
                          seq-local: [w270 _ _ _ _] -> [_ w283 _ _ _]
                          seq-local: [_ w284 _ _ _] -> [_ _ w296 _ _]
                          seq-local: [_ _ w295 _ _] -> [_ _ _ w309 _]
                          seq-local: [_ _ _ w305 _] -> [_ _ _ _ w321]
                          tunnel: w266 -> [w278 _ _ _ _]
                          tunnel: [_ _ _ _ w318] -> w265
                          frame #0 {
                            n79 = Unbundle(w278) -> ("SR830 VISA Name"=w277:refnum<visa-resource-name>, "SR830 Error"=w276:errorcluster)  [unwired: 6 out]
                            n80 = VISA Write(VISA resource name=w277, write buffer="FREQ?", error in (no error)=w276) -> (VISA resource name out=w279:refnum<visa-resource-name>, error out=w275:errorcluster)  [unwired: 1 out]
                            n81 = VISA Read(VISA resource name=w279, byte count=u32 50, error in (no error)=w275) -> (VISA resource name out=w273:refnum<visa-resource-name>, read buffer=w269:string, error out=w274:errorcluster)  [unwired: 1 out]
                            n82 = Bundle(cluster=w278, "SR830 VISA Name"=w273, "SR830 Error"=w274) -> (w270:T7)  [unwired: 6 in]
                            n83 = Scan Value(string=w269, format string="%f") -> (value=→"Ref. Freq.":dbl)  [unwired: 1 in, 1 out]
                          }
                          frame #1 {
                            n84 = Unbundle(w283) -> ("SR830 VISA Name"=w291:refnum<visa-resource-name>, "SR830 Error"=w290:errorcluster)  [unwired: 6 out]
                            n85 = VISA Write(VISA resource name=w291, write buffer="SLVL?", error in (no error)=w290) -> (VISA resource name out=w292:refnum<visa-resource-name>, error out=w289:errorcluster)  [unwired: 1 out]
                            n86 = VISA Read(VISA resource name=w292, byte count=u32 50, error in (no error)=w289) -> (VISA resource name out=w287:refnum<visa-resource-name>, read buffer=w281:string, error out=w288:errorcluster)  [unwired: 1 out]
                            n87 = Bundle(cluster=w283, "SR830 VISA Name"=w287, "SR830 Error"=w288) -> (w284:T7)  [unwired: 6 in]
                            n88 = Scan Value(string=w281, format string="%f") -> (value=w280:dbl)  [unwired: 1 in, 1 out]
                            "Ref. Amp." <- w280
                            n89 = local write "Ref\nVoltage (V)"(w280) -> ()
                          }
                          frame #2 {
                            n90 = Unbundle(w296) -> ("SR830 VISA Name"=w303:refnum<visa-resource-name>, "SR830 Error"=w302:errorcluster)  [unwired: 6 out]
                            n91 = VISA Write(VISA resource name=w303, write buffer="HARM?", error in (no error)=w302) -> (VISA resource name out=w304:refnum<visa-resource-name>, error out=w301:errorcluster)  [unwired: 1 out]
                            n92 = VISA Read(VISA resource name=w304, byte count=u32 50, error in (no error)=w301) -> (VISA resource name out=w299:refnum<visa-resource-name>, read buffer=w294:string, error out=w300:errorcluster)  [unwired: 1 out]
                            n93 = Decimal String To Number(string=w294) -> (number=→"Ref. Harm.":i32)  [unwired: 2 in, 1 out]
                            n94 = Bundle(cluster=w296, "SR830 VISA Name"=w299, "SR830 Error"=w300) -> (w295:T7)  [unwired: 6 in]
                          }
                          frame #3 {
                            n95 = Unbundle(w309) -> ("SR830 VISA Name"=w316:refnum<visa-resource-name>, "SR830 Error"=w315:errorcluster)  [unwired: 6 out]
                            n96 = VISA Write(VISA resource name=w316, write buffer="PHAS?", error in (no error)=w315) -> (VISA resource name out=w317:refnum<visa-resource-name>, error out=w314:errorcluster)  [unwired: 1 out]
                            n97 = VISA Read(VISA resource name=w317, byte count=u32 50, error in (no error)=w314) -> (VISA resource name out=w312:refnum<visa-resource-name>, read buffer=w307:string, error out=w313:errorcluster)  [unwired: 1 out]
                            n98 = Bundle(cluster=w309, "SR830 VISA Name"=w312, "SR830 Error"=w313) -> (w305:T7)  [unwired: 6 in]
                            n99 = Scan Value(string=w307, format string="%f") -> (value=→"Ref. Phase":dbl)  [unwired: 1 in, 1 out]
                          }
                          frame #4 {
                            n100 = Unbundle(w321) -> ("SR830 VISA Name"=w328:refnum<visa-resource-name>, "SR830 Error"=w327:errorcluster)  [unwired: 6 out]
                            n101 = VISA Write(VISA resource name=w328, write buffer="FMOD?", error in (no error)=w327) -> (VISA resource name out=w329:refnum<visa-resource-name>, error out=w326:errorcluster)  [unwired: 1 out]
                            n102 = VISA Read(VISA resource name=w329, byte count=u32 50, error in (no error)=w326) -> (VISA resource name out=w324:refnum<visa-resource-name>, read buffer=w320:string, error out=w325:errorcluster)  [unwired: 1 out]
                            n103 = Bundle(cluster=w321, "SR830 VISA Name"=w324, "SR830 Error"=w325) -> (w318:T7)  [unwired: 6 in]
                            n104 = Decimal String To Number(string=w320) -> (number=→"Trigger Source":i32)  [unwired: 2 in, 1 out]
                          }
                        }
                      }
                      frame #1 {
                        # "SR830 Display Channel1&2 Info"
                        n105 = stacked-sequence {
                          seq-local: [w336 _] -> [_ w351]
                          tunnel: w331 -> [w344 _]
                          tunnel: [_ w350] -> w330
                          frame #0 {
                            n106 = Unbundle(w344) -> ("SR830 VISA Name"=w343:refnum<visa-resource-name>, "SR830 Error"=w342:errorcluster)  [unwired: 6 out]
                            n107 = VISA Write(VISA resource name=w343, write buffer="DDEF? 1", error in (no error)=w342) -> (VISA resource name out=w345:refnum<visa-resource-name>, error out=w341:errorcluster)  [unwired: 1 out]
                            n108 = VISA Read(VISA resource name=w345, byte count=u32 50, error in (no error)=w341) -> (VISA resource name out=w339:refnum<visa-resource-name>, read buffer=w334:string, error out=w340:errorcluster)  [unwired: 1 out]
                            n109 = Bundle(cluster=w344, "SR830 VISA Name"=w339, "SR830 Error"=w340) -> (w336:T7)  [unwired: 6 in]
                            n110 = Decimal String To Number(string=w334) -> (number=→"Channel 1 Display":i32)  [unwired: 2 in, 1 out]
                            n111 = Decimal String To Number(string=w334, offset=2) -> (number=→"Channel 1 Display With Ratio":i32)  [unwired: 1 in, 1 out]
                          }
                          frame #1 {
                            n112 = Unbundle(w351) -> ("SR830 VISA Name"=w358:refnum<visa-resource-name>, "SR830 Error"=w357:errorcluster)  [unwired: 6 out]
                            n113 = VISA Write(VISA resource name=w358, write buffer="DDEF? 2", error in (no error)=w357) -> (VISA resource name out=w359:refnum<visa-resource-name>, error out=w356:errorcluster)  [unwired: 1 out]
                            n114 = VISA Read(VISA resource name=w359, byte count=u32 50, error in (no error)=w356) -> (VISA resource name out=w354:refnum<visa-resource-name>, read buffer=w348:string, error out=w355:errorcluster)  [unwired: 1 out]
                            n115 = Bundle(cluster=w351, "SR830 VISA Name"=w354, "SR830 Error"=w355) -> (w350:T7)  [unwired: 6 in]
                            n116 = Decimal String To Number(string=w348) -> (number=→"Channel 2 Display":i32)  [unwired: 2 in, 1 out]
                            n117 = Decimal String To Number(string=w348, offset=2) -> (number=→"Channel 2 Display With Ratio":i32)  [unwired: 1 in, 1 out]
                          }
                        }
                      }
                      frame #2 {
                        # "SR830 Signal Input Info"
                        n118 = stacked-sequence {
                          seq-local: [w364 _ _ _] -> [_ w377 _ _]
                          seq-local: [_ w376 _ _] -> [_ _ w389 _]
                          seq-local: [_ _ w388 _] -> [_ _ _ w400]
                          tunnel: w361 -> [w372 _ _ _]
                          tunnel: [_ _ _ w401] -> w360
                          frame #0 {
                            n119 = Unbundle(w372) -> ("SR830 VISA Name"=w371:refnum<visa-resource-name>, "SR830 Error"=w370:errorcluster)  [unwired: 6 out]
                            n120 = VISA Write(VISA resource name=w371, write buffer="ISRC?", error in (no error)=w370) -> (VISA resource name out=w373:refnum<visa-resource-name>, error out=w369:errorcluster)  [unwired: 1 out]
                            n121 = VISA Read(VISA resource name=w373, byte count=u32 50, error in (no error)=w369) -> (VISA resource name out=w367:refnum<visa-resource-name>, read buffer=w363:string, error out=w368:errorcluster)  [unwired: 1 out]
                            n122 = Bundle(cluster=w372, "SR830 VISA Name"=w367, "SR830 Error"=w368) -> (w364:T7)  [unwired: 6 in]
                            n123 = Decimal String To Number(string=w363) -> (number=→"Input Connection":i32)  [unwired: 2 in, 1 out]
                          }
                          frame #1 {
                            n124 = Unbundle(w377) -> ("SR830 VISA Name"=w384:refnum<visa-resource-name>, "SR830 Error"=w383:errorcluster)  [unwired: 6 out]
                            n125 = VISA Write(VISA resource name=w384, write buffer="ICPL?", error in (no error)=w383) -> (VISA resource name out=w385:refnum<visa-resource-name>, error out=w382:errorcluster)  [unwired: 1 out]
                            n126 = VISA Read(VISA resource name=w385, byte count=u32 50, error in (no error)=w382) -> (VISA resource name out=w380:refnum<visa-resource-name>, read buffer=w375:string, error out=w381:errorcluster)  [unwired: 1 out]
                            n127 = Decimal String To Number(string=w375) -> (number=→"Input Coupling":i32)  [unwired: 2 in, 1 out]
                            n128 = Bundle(cluster=w377, "SR830 VISA Name"=w380, "SR830 Error"=w381) -> (w376:T7)  [unwired: 6 in]
                          }
                          frame #2 {
                            n129 = Unbundle(w389) -> ("SR830 VISA Name"=w396:refnum<visa-resource-name>, "SR830 Error"=w395:errorcluster)  [unwired: 6 out]
                            n130 = VISA Write(VISA resource name=w396, write buffer="IGND?", error in (no error)=w395) -> (VISA resource name out=w397:refnum<visa-resource-name>, error out=w394:errorcluster)  [unwired: 1 out]
                            n131 = VISA Read(VISA resource name=w397, byte count=u32 50, error in (no error)=w394) -> (VISA resource name out=w392:refnum<visa-resource-name>, read buffer=w387:string, error out=w393:errorcluster)  [unwired: 1 out]
                            n132 = Bundle(cluster=w389, "SR830 VISA Name"=w392, "SR830 Error"=w393) -> (w388:T7)  [unwired: 6 in]
                            n133 = Decimal String To Number(string=w387) -> (number=→"Input Shield Grounding":i32)  [unwired: 2 in, 1 out]
                          }
                          frame #3 {
                            n134 = Unbundle(w400) -> ("SR830 VISA Name"=w408:refnum<visa-resource-name>, "SR830 Error"=w407:errorcluster)  [unwired: 6 out]
                            n135 = VISA Write(VISA resource name=w408, write buffer="ILIN?", error in (no error)=w407) -> (VISA resource name out=w409:refnum<visa-resource-name>, error out=w406:errorcluster)  [unwired: 1 out]
                            n136 = VISA Read(VISA resource name=w409, byte count=u32 50, error in (no error)=w406) -> (VISA resource name out=w404:refnum<visa-resource-name>, read buffer=w398:string, error out=w405:errorcluster)  [unwired: 1 out]
                            n137 = Decimal String To Number(string=w398) -> (number=→"Input Notch Filter":i32)  [unwired: 2 in, 1 out]
                            n138 = Bundle(cluster=w400, "SR830 VISA Name"=w404, "SR830 Error"=w405) -> (w401:T7)  [unwired: 6 in]
                          }
                        }
                      }
                      frame #3 {
                        # "SR830 Measurement Settings"
                        n139 = stacked-sequence {
                          seq-local: [w414 _ _ _ _] -> [_ w427 _ _ _]
                          seq-local: [_ w426 _ _ _] -> [_ _ w439 _ _]
                          seq-local: [_ _ w438 _ _] -> [_ _ _ w451 _]
                          seq-local: [_ _ _ w448 _] -> [_ _ _ _ w462]
                          tunnel: w411 -> [w422 _ _ _ _]
                          tunnel: [_ _ _ _ w461] -> w410
                          frame #0 {
                            n140 = Unbundle(w422) -> ("SR830 VISA Name"=w421:refnum<visa-resource-name>, "SR830 Error"=w420:errorcluster)  [unwired: 6 out]
                            n141 = VISA Write(VISA resource name=w421, write buffer="SENS?", error in (no error)=w420) -> (VISA resource name out=w423:refnum<visa-resource-name>, error out=w419:errorcluster)  [unwired: 1 out]
                            n142 = VISA Read(VISA resource name=w423, byte count=u32 50, error in (no error)=w419) -> (VISA resource name out=w417:refnum<visa-resource-name>, read buffer=w413:string, error out=w418:errorcluster)  [unwired: 1 out]
                            n143 = Bundle(cluster=w422, "SR830 VISA Name"=w417, "SR830 Error"=w418) -> (w414:T7)  [unwired: 6 in]
                            n144 = Decimal String To Number(string=w413) -> (number=→"Sensitivity":i32)  [unwired: 2 in, 1 out]
                          }
                          frame #1 {
                            n145 = Unbundle(w427) -> ("SR830 VISA Name"=w434:refnum<visa-resource-name>, "SR830 Error"=w433:errorcluster)  [unwired: 6 out]
                            n146 = VISA Write(VISA resource name=w434, write buffer="OFLT?", error in (no error)=w433) -> (VISA resource name out=w435:refnum<visa-resource-name>, error out=w432:errorcluster)  [unwired: 1 out]
                            n147 = VISA Read(VISA resource name=w435, byte count=u32 50, error in (no error)=w432) -> (VISA resource name out=w430:refnum<visa-resource-name>, read buffer=w425:string, error out=w431:errorcluster)  [unwired: 1 out]
                            n148 = Decimal String To Number(string=w425) -> (number=→"Time Constant":i32)  [unwired: 2 in, 1 out]
                            n149 = Bundle(cluster=w427, "SR830 VISA Name"=w430, "SR830 Error"=w431) -> (w426:T7)  [unwired: 6 in]
                          }
                          frame #2 {
                            n150 = Unbundle(w439) -> ("SR830 VISA Name"=w446:refnum<visa-resource-name>, "SR830 Error"=w445:errorcluster)  [unwired: 6 out]
                            n151 = VISA Write(VISA resource name=w446, write buffer="RMOD?", error in (no error)=w445) -> (VISA resource name out=w447:refnum<visa-resource-name>, error out=w444:errorcluster)  [unwired: 1 out]
                            n152 = VISA Read(VISA resource name=w447, byte count=u32 50, error in (no error)=w444) -> (VISA resource name out=w442:refnum<visa-resource-name>, read buffer=w437:string, error out=w443:errorcluster)  [unwired: 1 out]
                            n153 = Decimal String To Number(string=w437) -> (number=→"Dynamic Reserve":i32)  [unwired: 2 in, 1 out]
                            n154 = Bundle(cluster=w439, "SR830 VISA Name"=w442, "SR830 Error"=w443) -> (w438:T7)  [unwired: 6 in]
                          }
                          frame #3 {
                            n155 = Unbundle(w451) -> ("SR830 VISA Name"=w458:refnum<visa-resource-name>, "SR830 Error"=w457:errorcluster)  [unwired: 6 out]
                            n156 = VISA Write(VISA resource name=w458, write buffer="OFSL?", error in (no error)=w457) -> (VISA resource name out=w459:refnum<visa-resource-name>, error out=w456:errorcluster)  [unwired: 1 out]
                            n157 = VISA Read(VISA resource name=w459, byte count=u32 50, error in (no error)=w456) -> (VISA resource name out=w454:refnum<visa-resource-name>, read buffer=w450:string, error out=w455:errorcluster)  [unwired: 1 out]
                            n158 = Decimal String To Number(string=w450) -> (number=→"Low Pass Filter Slope":i32)  [unwired: 2 in, 1 out]
                            n159 = Bundle(cluster=w451, "SR830 VISA Name"=w454, "SR830 Error"=w455) -> (w448:T7)  [unwired: 6 in]
                          }
                          frame #4 {
                            n160 = Unbundle(w462) -> ("SR830 VISA Name"=w470:refnum<visa-resource-name>, "SR830 Error"=w469:errorcluster)  [unwired: 6 out]
                            n161 = VISA Write(VISA resource name=w470, write buffer="SYNC?", error in (no error)=w469) -> (VISA resource name out=w471:refnum<visa-resource-name>, error out=w468:errorcluster)  [unwired: 1 out]
                            n162 = VISA Read(VISA resource name=w471, byte count=u32 50, error in (no error)=w468) -> (VISA resource name out=w466:refnum<visa-resource-name>, read buffer=w463:string, error out=w467:errorcluster)  [unwired: 1 out]
                            n163 = Decimal String To Number(string=w463) -> (number=→"Sync Filter Enabled":i32)  [unwired: 2 in, 1 out]
                            n164 = Bundle(cluster=w462, "SR830 VISA Name"=w466, "SR830 Error"=w467) -> (w461:T7)  [unwired: 6 in]
                          }
                        }
                      }
                      frame #4 {
                        # "SR830 Channel Measurements"
                        n165 = Unbundle(w475) -> ("SR830 VISA Name"=w479:refnum<visa-resource-name>, "SR830 Error"=w478:errorcluster)  [unwired: 6 out]
                        n166 = call-poly <instrlib>:"Read.vi"("error in (no error)"=w478, "VISA resource name"=w479) -> ("error out"=w476:errorcluster, "Parameter Values"=w480:T9, "VISA resource name out"=w477:refnum<visa-resource-name>)  [unwired: 7 in]
                        n167 = Bundle(cluster=w475, "SR830 VISA Name"=w477, "SR830 Error"=w476) -> (w474:T7)  [unwired: 6 in]
                        n168 = Unbundle(w480) -> ("Channel 1 Display"=w473:dbl, "Channel 2 Display"=w472:dbl)  [unwired: 9 out]
                        n169 = local write "Channel 1\nMeasurement"(w473) -> ()
                        n170 = local write "Channel 2\nMeasurement"(w472) -> ()
                      }
                    }
                  }
                }
              }
              event User Event; "Aquire SR830 GS": Mouse Up {
                n171 = event-data() -> ()  [unwired: 1 in, 3 out]
                n172 = local read "Keithley 24XX Initialized / Off"() -> (w484:bool)
                n173 = case shown="True" w484 {
                  tunnel: w483 -> [w485 w487]
                  tunnel: [w485 w486] -> w482
                  frame False {
                  }
                  frame True {
                    n174 = stacked-sequence {
                      seq-local: [w489 _] -> [_ w547]
                      tunnel: [_ w548] -> w486
                      tunnel: w487 -> [w488 _]
                      frame #0 {
                        # "Check current output / source state"
                        n175 = stacked-sequence {
                          seq-local: [w490 _ _ _] -> [_ w505 _ _]
                          seq-local: [_ w504 _ _] -> [_ _ w515 _]
                          seq-local: [_ _ w514 _] -> [_ _ _ w540]
                          tunnel: w488 -> [w502 _ _ _]
                          tunnel: [_ _ _ w527] -> w489
                          frame #0 {
                            n176 = Unbundle(w502) -> ("Keithley 24XX VISA Name"=w498:refnum<visa-resource-name>, "Keithley 24XX Error"=w497:errorcluster)  [unwired: 6 out]
                            n177 = VISA Write(VISA resource name=w498, write buffer=":OUTP:STAT?", error in (no error)=w497) -> (VISA resource name out=w496:refnum<visa-resource-name>, error out=w501:errorcluster)  [unwired: 1 out]
                            n178 = VISA Read(VISA resource name=w496, byte count=u32 50, error in (no error)=w501) -> (VISA resource name out=w494:refnum<visa-resource-name>, read buffer=w493:string, error out=w495:errorcluster)  [unwired: 1 out]
                            n179 = Bundle(cluster=w502, "Keithley 24XX VISA Name"=w494, "Keithley 24XX Error"=w495) -> (w490:T7)  [unwired: 6 in]
                            n180 = Decimal String To Number(string=w493) -> (number=w492:i32)  [unwired: 2 in, 1 out]
                            n181 = Not Equal To 0?(x=w492) -> (x != 0?=→"Output On/Off":bool)
                          }
                          frame #1 {
                            n182 = Unbundle(w505) -> ("Keithley 24XX VISA Name"=w510:refnum<visa-resource-name>, "Keithley 24XX Error"=w509:errorcluster)  [unwired: 6 out]
                            n183 = VISA Write(VISA resource name=w510, write buffer=":OUTP:SMOD?", error in (no error)=w509) -> (VISA resource name out=w508:refnum<visa-resource-name>, error out=w513:errorcluster)  [unwired: 1 out]
                            n184 = VISA Read(VISA resource name=w508, byte count=u32 50, error in (no error)=w513) -> (VISA resource name out=w506:refnum<visa-resource-name>, read buffer=→"Output Impedence Mode":string, error out=w507:errorcluster)  [unwired: 1 out]
                            n185 = Bundle(cluster=w505, "Keithley 24XX VISA Name"=w506, "Keithley 24XX Error"=w507) -> (w504:T7)  [unwired: 6 in]
                          }
                          frame #2 {
                            n186 = Unbundle(w515) -> ("Keithley 24XX VISA Name"=w521:refnum<visa-resource-name>, "Keithley 24XX Error"=w520:errorcluster)  [unwired: 6 out]
                            n187 = VISA Write(VISA resource name=w521, write buffer=":ROUT:TERM?", error in (no error)=w520) -> (VISA resource name out=w519:refnum<visa-resource-name>, error out=w524:errorcluster)  [unwired: 1 out]
                            n188 = VISA Read(VISA resource name=w519, byte count=u32 50, error in (no error)=w524) -> (VISA resource name out=w517:refnum<visa-resource-name>, read buffer=→"Front / Rear Terminals":string, error out=w518:errorcluster)  [unwired: 1 out]
                            n189 = Bundle(cluster=w515, "Keithley 24XX VISA Name"=w517, "Keithley 24XX Error"=w518) -> (w514:T7)  [unwired: 6 in]
                          }
                          frame #3 {
                            n190 = Unbundle(w540) -> ("Keithley 24XX VISA Name"=w543:refnum<visa-resource-name>, "Keithley 24XX Error"=w542:errorcluster)  [unwired: 6 out]
                            n191 = VISA Write(VISA resource name=w543, write buffer=":SOUR:FUNC:MODE?", error in (no error)=w542) -> (VISA resource name out=w541:refnum<visa-resource-name>, error out=w546:errorcluster)  [unwired: 1 out]
                            n192 = VISA Read(VISA resource name=w541, byte count=u32 50, error in (no error)=w546) -> (VISA resource name out=w534:refnum<visa-resource-name>, read buffer=w526:string, error out=w535:errorcluster)  [unwired: 1 out]
                            "Source Mode:" <- w526
                            n193 = call <vilib>:"Trim Whitespace.vi"("string"=w526) -> ("trimmed string"=w525:string)  [unwired: 1 in]
                            n194 = Concatenate Strings(":SOUR:" ("string"), w525, ":LEV:IMM:AMPL?" ("string")) -> (w531:string)
                            n195 = VISA Write(VISA resource name=w534, write buffer=w531, error in (no error)=w535) -> (VISA resource name out=w537:refnum<visa-resource-name>, error out=w539:errorcluster)  [unwired: 1 out]
                            n196 = VISA Read(VISA resource name=w537, byte count=u32 50, error in (no error)=w539) -> (read buffer=w529:string, error out=w536:errorcluster)  [unwired: 2 out]
                            n197 = Bundle(cluster=w540, "Keithley 24XX Error"=w536) -> (w527:T7)  [unwired: 7 in]
                            n198 = Scan Value(string=w529, format string="%f") -> (value=→"Source Amplitude":dbl)  [unwired: 1 in, 1 out]
                          }
                        }
                      }
                      frame #1 {
                        # "Check the sense state"
                        n199 = stacked-sequence {
                          seq-local: [w553 _ _] -> [_ w564 _]
                          seq-local: [_ w563 _] -> [_ _ w574]
                          tunnel: [_ _ w573] -> w548
                          tunnel: w547 -> [w551 _ _]
                          frame #0 {
                            n200 = Unbundle(w551) -> ("Keithley 24XX VISA Name"=w550:refnum<visa-resource-name>, "Keithley 24XX Error"=w549:errorcluster)  [unwired: 6 out]
                            n201 = VISA Write(VISA resource name=w550, write buffer=":SYST:RSEN?", error in (no error)=w549) -> (VISA resource name out=w557:refnum<visa-resource-name>, error out=w560:errorcluster)  [unwired: 1 out]
                            n202 = VISA Read(VISA resource name=w557, byte count=u32 50, error in (no error)=w560) -> (VISA resource name out=w555:refnum<visa-resource-name>, read buffer=w554:string, error out=w556:errorcluster)  [unwired: 1 out]
                            n203 = Bundle(cluster=w551, "Keithley 24XX VISA Name"=w555, "Keithley 24XX Error"=w556) -> (w553:T7)  [unwired: 6 in]
                            n204 = Decimal String To Number(string=w554) -> (number=→"4 Probe Senseing":i32)  [unwired: 2 in, 1 out]
                          }
                          frame #1 {
                            n205 = Pick Line(multi-line string="VOLT\nCURR\nRES") -> ()  [unwired: 2 in, 1 out]
                            n206 = Match First String() -> ()  [unwired: 2 in, 2 out]
                            n207 = Unbundle(w564) -> ("Keithley 24XX VISA Name"=w569:refnum<visa-resource-name>, "Keithley 24XX Error"=w568:errorcluster)  [unwired: 6 out]
                            n208 = VISA Write(VISA resource name=w569, write buffer=":SENS:FUNC:ON?", error in (no error)=w568) -> (VISA resource name out=w567:refnum<visa-resource-name>, error out=w572:errorcluster)  [unwired: 1 out]
                            n209 = VISA Read(VISA resource name=w567, byte count=u32 50, error in (no error)=w572) -> (VISA resource name out=w565:refnum<visa-resource-name>, read buffer=→"Enabled Sensing\nFunctions":string, error out=w566:errorcluster)  [unwired: 1 out]
                            n210 = Bundle(cluster=w564, "Keithley 24XX VISA Name"=w565, "Keithley 24XX Error"=w566) -> (w563:T7)  [unwired: 6 in]
                          }
                          frame #2 {
                            n211 = Unbundle(w574) -> ("Keithley 24XX VISA Name"=w580:refnum<visa-resource-name>, "Keithley 24XX Error"=w579:errorcluster)  [unwired: 6 out]
                            n212 = VISA Write(VISA resource name=w580, write buffer=":SENS:CURR:RANG:AUTO:ULIM?", error in (no error)=w579) -> (VISA resource name out=w578:refnum<visa-resource-name>, error out=w583:errorcluster)  [unwired: 1 out]
                            n213 = VISA Read(VISA resource name=w578, byte count=u32 50, error in (no error)=w583) -> (VISA resource name out=w576:refnum<visa-resource-name>, read buffer=→"Sensing Current Upper Limit":string, error out=w577:errorcluster)  [unwired: 1 out]
                            n214 = Bundle(cluster=w574, "Keithley 24XX VISA Name"=w576, "Keithley 24XX Error"=w577) -> (w573:T7)  [unwired: 6 in]
                          }
                        }
                      }
                    }
                  }
                }
              }
              event User Event {
                n215 = event-data() -> ()  [unwired: 1 in, 4 out]
              }
              event User Event {
                n216 = event-data() -> ()  [unwired: 1 in, 4 out]
              }
              event "Program Selection": Value Change {
                n217 = event-data() -> ("NewVal"=w590:T5)  [unwired: 1 in, 5 out]
                n218 = case shown="\"Ramp Ref Voltage\"" w590 {
                  frame "4 Probe Gated Measurement", Default {
                    (unwired) T6."4 Probe Meas. Settings" ("SR830 Settings")
                    n219 = local read "SR830 Settings"() -> ()  [unwired: 1 in]
                  }
                  frame "Ramp Gate Voltage" {
                    (unwired) T6."Ramp Ref. Voltage" ("SR830 Settings")
                    n220 = local read "SR830 Settings"() -> ()  [unwired: 1 in]
                  }
                  frame "Ramp Ref Voltage" {
                  }
                }
              }
              event "Run Program": Mouse Up {
                n221 = event-data() -> ()  [unwired: 1 in, 8 out]
                n222 = local read "Program Selection"() -> (w593:T5)
                n223 = case shown="\"Ramp Ref Voltage\"" w593 {
                  tunnel: w595 -> [w599 w604 w607]
                  tunnel: [w598 w603 w606] -> w594
                  tunnel: "Program Iterations" -> [w597 _ _]
                  tunnel: [T3."Running single meas." T3."Running single meas." T3."Running single meas."] -> w591
                  frame "4 Probe Gated Measurement", Default {
                    n224 = Bundle(cluster=w599, "MeasurementsRemaining"=w597, "TotalMeasurements"=w597) -> (w598:T7)  [unwired: 6 in]
                  }
                  frame "Ramp Gate Voltage" {
                    n225 = Bundle(cluster=w604, "MeasurementsRemaining"=1, "TotalMeasurements"=1) -> (w603:T7)  [unwired: 6 in]
                  }
                  frame "Ramp Ref Voltage" {
                    n226 = Bundle(cluster=w607, "MeasurementsRemaining"=1, "TotalMeasurements"=1) -> (w606:T7)  [unwired: 6 in]
                  }
                }
              }
              event "Update SR830 GS": Mouse Up {
                n227 = event-data() -> ()  [unwired: 1 in, 8 out]
                n228 = local read "SR830 Initialized / Off"() -> (w617:bool)
                n229 = Unbundle(w615) -> ("SR830 VISA Name"=w610:refnum<visa-resource-name>, "SR830 Error"=w611:errorcluster)  [unwired: 6 out]
                n230 = case shown="True" w617 {
                  tunnel: [w619 w630] -> w614
                  tunnel: [w618 w631] -> w613
                  tunnel: w611 -> [w618 w628]
                  tunnel: w610 -> [w619 w629]
                  frame False {
                  }
                  frame True {
                    n231 = flat-sequence {
                      tunnel: w629 -> [w637]
                      tunnel: w628 -> [w636]
                      tunnel: [w635] -> w626
                      tunnel: [w634] -> w624
                      tunnel: ["Sine Ref Amplitude (V)"] -> w622
                      tunnel: [w632] -> w621
                      tunnel: [w648] -> w627
                      tunnel: w626 -> [w648]
                      tunnel: [w647] -> w625
                      tunnel: w624 -> [w647]
                      tunnel: [w645] -> w623
                      tunnel: w622 -> [w645]
                      tunnel: w621 -> [w646]
                      tunnel: [w644] -> w620
                      tunnel: [w672] -> w631
                      tunnel: [w671] -> w630
                      tunnel: w627 -> [w670]
                      tunnel: w625 -> [w669]
                      tunnel: w623 -> [w668]
                      tunnel: w620 -> [w667]
                      frame #0 {
                        n232 = VISA Write(VISA resource name=w637, write buffer="SLVL?", error in (no error)=w636) -> (VISA resource name out=w641:refnum<visa-resource-name>, error out=w643:errorcluster)  [unwired: 1 out]
                        n233 = VISA Read(VISA resource name=w641, byte count=u32 50, error in (no error)=w643) -> (VISA resource name out=w634:refnum<visa-resource-name>, read buffer=w642:string, error out=w635:errorcluster)  [unwired: 1 out]
                        n234 = Scan Value(string=w642, format string="%f") -> (value=w632:dbl)  [unwired: 1 in, 1 out]
                      }
                      frame #1 {
                        n235 = Not Equal?(x=w646, y=w645) -> (x != y?=w649:bool)
                        n236 = case shown="True" w649 {
                          tunnel: [TRUE ("T button?") w657] -> w644
                          tunnel: w646 -> [_ w652]
                          tunnel: w645 -> [_ w651]
                          frame False {
                          }
                          frame True {
                            w655 = "\r\n"
                            w653 = "\r\n"
                            n237 = Format Into String(format string="%f", initial string="Instrument Ref: ", w652) -> (resulting string=w659:string)  [unwired: 1 in, 1 out]
                            n238 = Format Into String(format string="%f", initial string="Specified Ref: ", w651) -> (resulting string=w658:string)  [unwired: 1 in, 1 out]
                            n239 = Concatenate Strings("Your specified output ref voltage doesn't match the detected reference voltage." ("message"), w653, w653, w659, w653, w658, w655, w655, "Are you sure you want to cause a jump?" ("string")) -> (w664:string)
                            n240 = Two Button Dialog(message=w664, 1:"No" ("F button name (\"Cancel\")"), 2:"Yep, jumping is fine." ("T button name (\"OK\")")) -> (T button?=w657:bool)
                          }
                        }
                      }
                      frame #2 {
                        n241 = case shown="False" w667 {
                          tunnel: [w674 w679] -> w672
                          tunnel: [w673 w678] -> w671
                          tunnel: w670 -> [w674 w677]
                          tunnel: w669 -> [w673 w676]
                          tunnel: w668 -> [_ w675]
                          frame False {
                          }
                          frame True {
                            w680 = u16 1 items=["Sine Zero Crossing", "TTL Rising Edge", "TTL Falling Edge"] ("External Reference Trigger (0: Sine Zero Crossing)")
                            w681 = u16 1 items=["External", "Internal"] ("Reference Source (1: Internal)")
                            n242 = call <instrlib>:"Configure Input Signal.vi"("Input Notch Filter (0: None)"="Input Notch Filter (0: None)", "Input Shield Grounding (0: Float)"="Input Shield Grounding", "error in (no error)"=w677, "Input Coupling (0: AC)"="Input Coupling", "Input Connection (0: Single-Ended Voltage)"="Input Connection", "VISA resource name"=w676) -> ("error out"=w688:errorcluster, "VISA resource name out"=w687:refnum<visa-resource-name>)  [unwired: 4 in]
                            n243 = call <instrlib>:"Configure Trigger.vi"("error in (no error)"=w688, "Trigger Source (0: Internal)"="Trigger Source", "VISA resource name"=w687) -> ()  [unwired: 7 in, 2 out]
                            n244 = call <instrlib>:"Configure Reference.vi"("Auto Phase (T: Enabled)"=FALSE, "Manual Phase (0 Degree)"="Manual Phase (Degree)", "Reference Source (1: Internal)"=w681, "Sine Output Amplitude (1 V)"=w675, "Detection Harmonic Number (1)"="Detection Harmonic Num.", "Internal Reference Frequency (1000 Hz)"="Internal Ref. Freq. (Hz)", "External Reference Trigger (0: Sine Zero Crossing)"=w680) -> ("VISA resource name out"=w686:refnum<visa-resource-name>, "error out"=w685:errorcluster)  [unwired: 7 in]
                            n245 = call <instrlib>:"Configure Filter.vi"("Enable Sync Filter (F: Disable)"="Sync Filter Enabled", "error in (no error)"=w685, "Low Pass Filter Slope (1: 12dB/oct)"="Low Pass Filter Slope", "Time Constant (8: 100ms)"="Time Constant", "VISA resource name"=w686) -> ("error out"=w683:errorcluster, "VISA resource name out"=w684:refnum<visa-resource-name>)  [unwired: 5 in]
                            n246 = call <instrlib>:"Configure Channel Display.vi"("Channel 2 Display With Ratio (0: None)"="Channel 2 Display With Ratio", "Channel 2 Display  (0: Y)"="Channel 2 Display", "error in (no error)"=w683, "Channel 1 Display With Ratio (0: None)"="Channel 1 Display With Ratio", "Channel 1 Display (0: X)"="Channel 1 Display", "VISA resource name"=w684) -> ("error out"=w701:errorcluster, "VISA resource name out"=w700:refnum<visa-resource-name>)  [unwired: 4 in]
                            n247 = call <instrlib>:"Configure Sensitivity and Reserve.vi"("error in (no error)"=w701, "Sensitivity (-1: Auto gain)"="Sensitivity", "Dynamic Reserve (-1: Auto Reserve)"="Dynamic Reserve", "VISA resource name"=w700) -> ("error out"=w679:errorcluster, "VISA resource name out"=w678:refnum<visa-resource-name>)  [unwired: 6 in]
                          }
                        }
                      }
                    }
                  }
                }
                n248 = Bundle(cluster=w615, "SR830 VISA Name"=w614, "SR830 Error"=w613) -> (w616:T7)  [unwired: 6 in]
              }
              event "Update Keithley 24XX GS": Mouse Up {
                n249 = event-data() -> ()  [unwired: 1 in, 8 out]
                n250 = local read "Keithley 24XX Initialized / Off"() -> (w708:bool)
                n251 = Unbundle(w714) -> ("Keithley 24XX VISA Name"=w712:refnum<visa-resource-name>, "Keithley 24XX Error"=w711:errorcluster)  [unwired: 6 out]
                n252 = case shown="True" w708 {
                  tunnel: w712 -> [w717 w721]
                  tunnel: w711 -> [w716 w720]
                  tunnel: [w717 w719] -> w710
                  tunnel: [w716 w718] -> w709
                  frame False {
                  }
                  frame True {
                    n253 = flat-sequence {
                      tunnel: w720 -> [w727]
                      tunnel: w721 -> [w728]
                      tunnel: [w728] -> w726
                      tunnel: [w727] -> w725
                      tunnel: [w731] -> w724
                      tunnel: [w730] -> w723
                      tunnel: w726 -> [w731]
                      tunnel: w725 -> [w730]
                      tunnel: [w729] -> w722
                      tunnel: w724 -> [w753]
                      tunnel: w723 -> [w752]
                      tunnel: w722 -> [w751]
                      tunnel: [w750] -> w719
                      tunnel: [w749] -> w718
                      frame #0 {
                      }
                      frame #1 {
                        n254 = case shown="True" {
                          selector: _ -> [_ _]
                          tunnel: [TRUE ("T button?") w739] -> w729
                          tunnel: _ -> [_ w734]
                          tunnel: _ -> [_ w733]
                          frame False {
                          }
                          frame True {
                            w737 = "\r\n"
                            w735 = "\r\n"
                            n255 = Format Into String(format string="%f", initial string="Instrument Ref: ", w734) -> (resulting string=w741:string)  [unwired: 1 in, 1 out]
                            n256 = Format Into String(format string="%f", initial string="Specified Ref: ", w733) -> (resulting string=w740:string)  [unwired: 1 in, 1 out]
                            n257 = Concatenate Strings("Your specified output ref voltage doesn't match the detected reference voltage." ("message"), w735, w735, w741, w735, w740, w737, w737, "Are you sure you want to cause a jump?" ("string")) -> (w746:string)
                            n258 = Two Button Dialog(message=w746, 1:"No" ("F button name (\"Cancel\")"), 2:"Yep, jumping is fine." ("T button name (\"OK\")")) -> (T button?=w739:bool)
                          }
                        }
                      }
                      frame #2 {
                        n259 = case shown="True" w751 {
                          tunnel: w753 -> [w755 w787]
                          tunnel: w752 -> [w754 w786]
                          tunnel: [w755 w761] -> w750
                          tunnel: [w754 w760] -> w749
                          frame False {
                          }
                          frame True {
                            w774 = u16 2 items=["Volts", "Current", "Resistance"] ("Function (0: Volts)")
                            w775 = u16 1 items=["Volts", "Current", "Resistance"] ("Function (0: Volts)")
                            w777 = u16 0 items=["Volts", "Current", "Resistance"] ("Function (0: Volts)")
                            # "Set the source voltage to limit, rather than sensing."
                            n260 = call <instrlib>:"Enable Remote Sensing.vi"("error in (no error)"=w786, "Enable Remote Sensing (T: Enable)"="Remote Sensing (4 Wire)", "VISA resource name"=w787) -> ("error out"=w790:errorcluster, "VISA resource name out"=w791:refnum<visa-resource-name>)  [unwired: 7 in]
                            n261 = call <instrlib>:"Display Measurement.vi"("error in (no error)"=w790, "Displayed Measurement (0: Voltage)"="Displayed Measurement (0: Voltage)", "VISA resource name"=w791) -> ("error out"=w789:errorcluster, "VISA resource name out"=w788:refnum<visa-resource-name>)  [unwired: 7 in]
                            n262 = call <instrlib>:"Configure Measurement.vi"("Manual Range (1.0)"="Voltage Manual Range", "error in (no error)"=w789, "Enable Auto Range (T:Enable)"="Voltage Auto Range", "Function (0: Volts)"=w777, "VISA resource name"=w788) -> ("error out"=w764:errorcluster, "VISA resource name out"=w765:refnum<visa-resource-name>)  [unwired: 5 in]
                            n263 = Absolute Value() -> (abs(x)=w781:dbl)  [unwired: 1 in]
                            n264 = Absolute Value() -> (abs(x)=w782:dbl)  [unwired: 1 in]
                            n265 = Max & Min(x=w782, y=w781) -> (max(x,y)=w780:dbl)  [unwired: 1 out]
                            n266 = call <instrlib>:"Configure Measurement.vi"("Manual Range (1.0)"="Current Manual Range", "error in (no error)"=w764, "Enable Auto Range (T:Enable)"="Current Auto Range", "Function (0: Volts)"=w775, "VISA resource name"=w765) -> ("error out"=w762:errorcluster, "VISA resource name out"=w763:refnum<visa-resource-name>)  [unwired: 5 in]
                            n267 = Format Into String(initial string="SOUR:VOLT:RANG %g", w780) -> (resulting string=w766:string)  [unwired: 2 in, 1 out]
                            n268 = call <instrlib>:"Configure Measurement.vi"("Manual Range (1.0)"="Resistance Manual Range", "error in (no error)"=w762, "Enable Auto Range (T:Enable)"="Resistance Auto Range", "Function (0: Volts)"=w774, "VISA resource name"=w763) -> ("error out"=w776:errorcluster, "VISA resource name out"=w785:refnum<visa-resource-name>)  [unwired: 5 in]
                            n269 = VISA Write(write buffer=w766) -> ()  [unwired: 2 in, 3 out]
                            n270 = call <instrlib>:"Configure Output.vi"("Output Type  (0: Immediate)"="Output Type  (0: Immediate)", "Source Mode  (0: Voltage)"="Source Mode  (0: Voltage)", "error in (no error)"=w776, "Compliance  Level (0.1)"="Compliance  Level (0.1)", "Output Level (0)"="Output Level (0)", "VISA resource name"=w785) -> ("error out"=w783:errorcluster, "VISA resource name out"=w784:refnum<visa-resource-name>)  [unwired: 4 in]
                            n271 = call <instrlib>:"Enable Output.vi"("error in (no error)"=w783, "VISA resource name"=w784) -> ("error out"=w760:errorcluster, "VISA resource name out"=w761:refnum<visa-resource-name>)  [unwired: 8 in]
                          }
                        }
                      }
                    }
                  }
                }
                n272 = Bundle(cluster=w714, "Keithley 24XX VISA Name"=w710, "Keithley 24XX Error"=w709) -> (w713:T7)  [unwired: 6 in]
              }
              event "Num Steps", "Total Time (s)": Value Change {
                # "Calculate the step time and step size"
                n273 = event-data() -> ()  [unwired: 1 in, 6 out]
                n274 = local read "Total Time (s)"() -> (w800:dbl)
                n275 = local read "Num Steps"() -> (w796:i32)
                n276 = Divide(x=w800, y=w796) -> (x/y=→"Step Time (ms)":dbl)
                n277 = local read "Final Output Amplitude (V)"() -> (w798:dbl)
                n278 = local read "Start Output Amplitude (V)"() -> (w797:dbl)
                n279 = Subtract(x=w798, y=w797) -> (x-y=w795:dbl)
                n280 = Divide(x=w795, y=w796) -> (x/y=→"Step Size (V)":dbl)
              }
            }
          }
          frame #1 {
            # "Boolean: At least one resource initialized?"
            n281 = local read "Keithley 24XX Initialized / Off"() -> (w801:bool)
            n282 = local read "Lakeshore Initialized / Off"() -> (w802:bool)
            n283 = local read "SR830 Initialized / Off"() -> (w803:bool)
            n284 = Build Array(w802, w803, w801) -> (w806:bool[])
            n285 = Or Array Elements(Boolean array=w806) -> (logical OR=w807:bool)
            n286 = case shown="False" w807 {
              tunnel: [T3."Off" w809] -> w805
              tunnel: w804 -> [_ w809]
              frame False {
              }
              frame True {
              }
            }
          }
          frame #2 {
            # "Polling for each device, to measure"
            n287 = stacked-sequence {
              seq-local: [w816 _ _] -> [_ w869 _]
              seq-local: [_ w870 _] -> [_ _ w877]
              tunnel: w811 -> [w819 _ _]
              tunnel: w810 -> [_ _ w875]
              tunnel: w814 -> [w817 _ _]
              tunnel: [_ _ w876] -> w813
              tunnel: w812 -> [_ w867 _]
              frame #0 {
                # "SR830 Status Measurements"
                n288 = stacked-sequence {
                  seq-local: [w820 _ _ _] -> [_ w833 _ _]
                  seq-local: [_ w832 _ _] -> [_ _ w848 _]
                  seq-local: [_ _ w847 _] -> [_ _ _ w860]
                  tunnel: w817 -> [w825 _ _ _]
                  tunnel: [_ _ _ w857] -> w816
                  frame #0 {
                    n289 = Unbundle(w825) -> ("SR830 VISA Name"=w830:refnum<visa-resource-name>, "SR830 Error"=w829:errorcluster)  [unwired: 6 out]
                    n290 = VISA Write(VISA resource name=w830, write buffer="DDEF? 1", error in (no error)=w829) -> (VISA resource name out=w831:refnum<visa-resource-name>, error out=w828:errorcluster)  [unwired: 1 out]
                    n291 = VISA Read(VISA resource name=w831, byte count=u32 50, error in (no error)=w828) -> (VISA resource name out=w821:refnum<visa-resource-name>, read buffer=w824:string, error out=w822:errorcluster)  [unwired: 1 out]
                    n292 = Decimal String To Number(string=w824) -> (number=w823:i32)  [unwired: 2 in, 1 out]
                    n293 = Bundle(cluster=w825, "SR830 VISA Name"=w821, "SR830 Error"=w822) -> (w820:T7)  [unwired: 6 in]
                    n294 = local write "Channel 1 Display"(w823) -> ()
                  }
                  frame #1 {
                    n295 = Unbundle(w833) -> ("SR830 VISA Name"=w842:refnum<visa-resource-name>, "SR830 Error"=w841:errorcluster)  [unwired: 6 out]
                    n296 = VISA Write(VISA resource name=w842, write buffer="DDEF? 2", error in (no error)=w841) -> (VISA resource name out=w843:refnum<visa-resource-name>, error out=w840:errorcluster)  [unwired: 1 out]
                    n297 = VISA Read(VISA resource name=w843, byte count=u32 50, error in (no error)=w840) -> (VISA resource name out=w835:refnum<visa-resource-name>, read buffer=w837:string, error out=w836:errorcluster)  [unwired: 1 out]
                    n298 = Decimal String To Number(string=w837) -> (number=w834:i32)  [unwired: 2 in, 1 out]
                    n299 = Bundle(cluster=w833, "SR830 VISA Name"=w835, "SR830 Error"=w836) -> (w832:T7)  [unwired: 6 in]
                    n300 = local write "Channel 2 Display"(w834) -> ()
                  }
                  frame #2 {
                    (unwired) "%f" ("format string")
                    n301 = Unbundle(w848) -> ("SR830 VISA Name"=w855:refnum<visa-resource-name>, "SR830 Error"=w854:errorcluster)  [unwired: 6 out]
                    n302 = VISA Write(VISA resource name=w855, write buffer="SLVL?", error in (no error)=w854) -> (VISA resource name out=w856:refnum<visa-resource-name>, error out=w853:errorcluster)  [unwired: 1 out]
                    n303 = VISA Read(VISA resource name=w856, byte count=u32 50, error in (no error)=w853) -> (VISA resource name out=w851:refnum<visa-resource-name>, read buffer=w845:string, error out=w852:errorcluster)  [unwired: 1 out]
                    n304 = Bundle(cluster=w848, "SR830 VISA Name"=w851, "SR830 Error"=w852) -> (w847:T7)  [unwired: 6 in]
                    n305 = Scan Value(string=w845, format string="%f") -> (value=w844:dbl)  [unwired: 1 in, 1 out]
                    n306 = local write "Ref. Amp."(w844) -> ()
                    n307 = local write "Ref\nVoltage (V)"(w844) -> ()
                  }
                  frame #3 {
                    n308 = Unbundle(w860) -> ("SR830 VISA Name"=w864:refnum<visa-resource-name>, "SR830 Error"=w863:errorcluster)  [unwired: 6 out]
                    n309 = call-poly <instrlib>:"Read.vi"("error in (no error)"=w863, "VISA resource name"=w864) -> ("error out"=w861:errorcluster, "Parameter Values"=w865:T9, "VISA resource name out"=w862:refnum<visa-resource-name>)  [unwired: 7 in]
                    n310 = Unbundle(w865) -> ("Channel 1 Display"=w859:dbl, "Channel 2 Display"=w858:dbl)  [unwired: 9 out]
                    n311 = Bundle(cluster=w860, "SR830 VISA Name"=w862, "SR830 Error"=w861) -> (w857:T7)  [unwired: 6 in]
                    n312 = local write "Channel 1\nMeasurement"(w859) -> ()
                    n313 = local write "Channel 2\nMeasurement"(w858) -> ()
                  }
                }
                n314 = And(x=w819, y="Idle Measure\nSR830 Status") -> ()  [unwired: 1 out]
              }
              frame #1 {
                # "Keithley 24XX Idle Measurements"
                n315 = And(x=w867, y="Idle Measure \nKeithley 24XX\nStatus") -> (x .and. y?=w866:bool)
                n316 = case shown="True" w866 {
                  tunnel: w869 -> [w871 w872]
                  tunnel: [w871 w872] -> w870
                  frame False {
                  }
                  frame True {
                  }
                }
              }
              frame #2 {
                # "Lakeshore 366 Idle Measurements"
                n317 = And(x=w875, y="Idle Measure\nLakeShore 336 \nStatus") -> (x .and. y?=w873:bool)
                n318 = case shown="True" w873 {
                  frame False {
                  }
                  frame True {
                  }
                }
                n319 = Unbundle(w877) -> ()  [unwired: 8 out]
                n320 = Bundle(cluster=w877) -> (w876:T7)  [unwired: 8 in]
              }
            }
          }
        }
      }
      frame "Running single meas." {
        n321 = case shown="\"Ramp Ref Voltage\"" w880 {
          tunnel: [w882 w883 w886 w903] -> w879
          tunnel: w878 -> [w882 w883 w885 w903]
          frame "4 Probe Gated Measurement", Default {
          }
          frame "Ramp Gate Voltage" {
          }
          frame "Ramp Ref Voltage" {
            n322 = flat-sequence {
              tunnel: [w888] -> w884
              tunnel: w885 -> [w889]
              tunnel: [w891] -> w886
              tunnel: w884 -> [w890]
              frame #0 {
                n323 = control-ref of="Reference Voltage"() -> (w888:refnum<vi>)
                n324 = property class="WFChart (strict)"(reference=w888, "History Data"=cluster{u32, dbl}[] [] ("array of clusters")) -> ()  [unwired: 1 in, 2 out]
              }
              frame #1 {
                n325 = local read "Final Output Amplitude (V)"() -> (w900:dbl)
                n326 = local read "Start Output Amplitude (V)"() -> (w899:dbl)
                n327 = control-ref of="Ref Voltage (V)"() -> (w896:refnum<vi>)
                n328 = control-ref of="Ref. Amp."() -> (w898:refnum<vi>)
                n329 = local read "Total Time (s)"() -> (w901:dbl)
                n330 = local read "Num Steps"() -> (w902:i32)
                n331 = Build Array(w896, w898) -> (w897:refnum<vi>[])
                n332 = Unbundle(w889) -> ("SR830 VISA Name"=w892:refnum<visa-resource-name>, "SR830 Error"=w893:errorcluster)  [unwired: 6 out]
                n333 = call <userlib>:"SR830_Source_Ramp_Algorithm.vi"("Total Time (s)"=w901, "Number of Steps"=w902, "Ref Level To"=w900, "Ref Level From"=w899, "error in (no error)"=w893, "Waveform Chart Reference"=w890, "Voltage Display\nReference"=w897, "VISA resource name"=w892) -> ("error out"=w895:errorcluster, "VISA resource name out"=w894:refnum<visa-resource-name>)  [unwired: 2 in]
                n334 = call <vilib>:"Simple Error Handler.vi"("error in (no error)"=w895) -> ()  [unwired: 4 in, 5 out]
                n335 = Bundle(cluster=w889, "SR830 VISA Name"=w894, "SR830 Error"=w895) -> (w891:T7)  [unwired: 6 in]
              }
            }
          }
          frame "Extra Option" {
          }
        }
      }
      frame "Running multi meas." {
        n336 = Unbundle(w910) -> ("MeasurementsRemaining"=w906:i32)  [unwired: 7 out]
        n337 = Less Or Equal To 0?(x=w906) -> (x <= 0?=w909:bool)
        n338 = case shown="True" w909 {
          tunnel: w908 -> [w914 _]
          tunnel: [w914 T3."Idle | Waiting for event"] -> w907
          tunnel: w906 -> [w912 _]
          tunnel: [w911 0] -> w905
          frame False {
            n339 = Subtract(x=w912, y=1) -> (x-y=w911:i32)
          }
          frame True {
          }
        }
        n340 = Bundle(cluster=w910, "MeasurementsRemaining"=w905) -> (w904:T7)  [unwired: 7 in]
      }
      frame "Running continuous meas." {
      }
    }
    "VI State" <- w32
  }
  n341 = disable-structure shown="Disabled" {
    frame Disabled {
      w931 = 1.0 ("Manual Range (1.0)")
      w934 = u16 1 items=["Voltage", "Current", "Resistance"] ("Displayed Measurement (0: Voltage)")
      w938 = u16 2 items=["Volts", "Current", "Resistance"] ("Function (0: Volts)")
      w942 = u16 1 items=["Volts", "Current", "Resistance"] ("Function (0: Volts)")
      w944 = u16 0 items=["Volts", "Current", "Resistance"] ("Function (0: Volts)")
      # "Find numeric range of input High/Low voltages"
      # "Set Display to Current"
      # "Config V,I & R settings to auto range"
      n342 = call <instrlib>:"Enable Output.vi"() -> ()  [unwired: 10 in, 2 out]
      n343 = Scan Value(format string="%f") -> ()  [unwired: 2 in, 2 out]
      n344 = VISA Write(write buffer="SLVL?") -> (error out=w922:errorcluster)  [unwired: 2 in, 2 out]
      n345 = VISA Write(write buffer="ISRC?") -> (error out=w925:errorcluster)  [unwired: 2 in, 2 out]
      n346 = VISA Read(byte count=u32 50, error in (no error)=w922) -> ()  [unwired: 1 in, 4 out]
      n347 = VISA Read(byte count=u32 50, error in (no error)=w925) -> ()  [unwired: 1 in, 4 out]
      n348 = Absolute Value() -> (abs(x)=w929:dbl)  [unwired: 1 in]
      n349 = Absolute Value() -> (abs(x)=w928:dbl)  [unwired: 1 in]
      n350 = call <instrlib>:"Configure Measurement.vi"("Manual Range (1.0)"=w931, "Enable Auto Range (T:Enable)"=TRUE, "Function (0: Volts)"=w942) -> ("error out"=w940:errorcluster, "VISA resource name out"=w935:refnum<visa-resource-name>)  [unwired: 7 in]
      n351 = Max & Min(x=w929, y=w928) -> (max(x,y)=w927:dbl)  [unwired: 1 out]
      n352 = Format Into String(initial string="%.;SOUR:VOLT:RANG %g ", w927) -> (resulting string=w926:string)  [unwired: 2 in, 1 out]
      n353 = Decimal String To Number() -> ()  [unwired: 3 in, 2 out]
      n354 = VISA Write(write buffer=w926) -> ()  [unwired: 2 in, 3 out]
      n355 = call <instrlib>:"Configure Measurement.vi"("Manual Range (1.0)"=w931, "error in (no error)"=w940, "Enable Auto Range (T:Enable)"=TRUE, "Function (0: Volts)"=w938, "VISA resource name"=w935) -> ("error out"=w937:errorcluster, "VISA resource name out"=w936:refnum<visa-resource-name>)  [unwired: 5 in]
      n356 = call-poly <instrlib>:"Read.vi"() -> ()  [unwired: 9 in, 7 out]
      n357 = call <instrlib>:"Configure Output.vi"() -> ()  [unwired: 10 in, 2 out]
      n358 = call <instrlib>:"Configure Measurement.vi"("Manual Range (1.0)"=w931, "error in (no error)"=w937, "Enable Auto Range (T:Enable)"=TRUE, "Function (0: Volts)"=w944, "VISA resource name"=w936) -> ("error out"=w932:errorcluster, "VISA resource name out"=w933:refnum<visa-resource-name>)  [unwired: 5 in]
      n359 = call <instrlib>:"Display Measurement.vi"("error in (no error)"=w932, "Displayed Measurement (0: Voltage)"=w934, "VISA resource name"=w933) -> ()  [unwired: 7 in, 2 out]
    }
    frame Enabled {
    }
  }
  n360 = Not Equal?(x=T3."Off", y=w15) -> (x != y?=w14:bool)
  n361 = case shown="True" w14 {
    tunnel: w13 -> [_ w951]
    frame False {
    }
    frame True {
      n362 = Unbundle(w951) -> ("Lakeshore 366 VISA Name"=w950:refnum<visa-resource-name>, "Lakeshore Error"=w949:errorcluster, "Keithley 24XX VISA Name"=w948:refnum<visa-resource-name>, "Keithley 24XX Error"=w947:errorcluster, "SR830 VISA Name"=w946:refnum<visa-resource-name>, "SR830 Error"=w945:errorcluster)  [unwired: 2 out]
      n363 = flat-sequence {
        tunnel: w946 -> [w953]
        tunnel: w945 -> [w952]
        tunnel: w948 -> [w960]
        tunnel: w947 -> [w959]
        tunnel: w950 -> [w967]
        tunnel: w949 -> [w966]
        frame #0 {
          n364 = local read "SR830 Initialized / Off"() -> (w954:bool)
          n365 = case shown="True" w954 {
            tunnel: w953 -> [_ w957]
            tunnel: w952 -> [_ w956]
            frame False {
            }
            frame True {
              n366 = call <instrlib>:"Close.vi"("error in (no error)"=w956, "VISA resource name"=w957) -> ("error out"=w958:errorcluster)  [unwired: 9 in]
              n367 = local write "SR830 Initialized / Off"(FALSE ("SR830 Initialized / Off")) -> ()
              n368 = call <vilib>:"Simple Error Handler.vi"("error in (no error)"=w958) -> ()  [unwired: 4 in, 5 out]
            }
          }
        }
        frame #1 {
          n369 = local read "Keithley 24XX Initialized / Off"() -> (w961:bool)
          n370 = case shown="True" w961 {
            tunnel: w960 -> [_ w964]
            tunnel: w959 -> [_ w963]
            frame False {
            }
            frame True {
              n371 = call <instrlib>:"Close.vi"("error in (no error)"=w963, "VISA resource name"=w964) -> ("error out"=w965:errorcluster)  [unwired: 9 in]
              n372 = local write "Keithley 24XX Initialized / Off"(FALSE ("SR830 Initialized / Off")) -> ()
              n373 = call <vilib>:"Simple Error Handler.vi"("error in (no error)"=w965) -> ()  [unwired: 4 in, 5 out]
            }
          }
        }
        frame #2 {
          n374 = local read "Lakeshore Initialized / Off"() -> (w968:bool)
          n375 = case shown="True" w968 {
            tunnel: w967 -> [_ w971]
            tunnel: w966 -> [_ w970]
            frame False {
            }
            frame True {
              n376 = call <instrlib>:"Close.vi"("error in (no error)"=w970, "VISA resource name"=w971) -> ("error out"=w972:errorcluster)  [unwired: 9 in]
              n377 = local write "Lakeshore Initialized / Off"(FALSE ("SR830 Initialized / Off")) -> ()
              n378 = call <vilib>:"Simple Error Handler.vi"("error in (no error)"=w972) -> ()  [unwired: 4 in, 5 out]
            }
          }
        }
      }
    }
  }
  "Gate Voltage" <- w19
  "Resistance / Differential" <- w19
  "Reference Voltage" <- cluster{u32, dbl}[] [] ("array of clusters")
